vi "WS1050 36 DUT Reliability HD_Cycling Ver1.6.vi"() -> ()   [LabVIEW 2012]
uses:
  WS_VCAP Driver 029/Source/WSVCAP Shell/Type Defs/WSVCAP SHL I2C DUT Mask Mode Enum.ctl
  <vilib>/Utility/file.llb/Read From Spreadsheet File (DBL).vi
panel:
  out "VISA resource name out":refnum<visa-resource-name>="GPIB0::3::INSTR"
  out "error out 2":errorcluster={"status"=TRUE, "code"=-63192, "source"="niLvFpga_Open_PXI-7813R.vi"}
  in  "Reg1_Bit Cntrl":string[](array[string])=["01", "02", "04", "08", "10", "20", "40", "80", "03", "06", "0C", "D8", "33", "66", "CC", "07", "0E", "1C", "38", "70", "E0", "0F", "1E", "3C", "78", "F0", "1F", "3E", "7C", "F8", "3F", "7E", "FC", "7F", "FE", "FD", "FB", "F7", "EF", "DF", "BF", "7F", "FC", "F9", "F3", "E7", "CF", "9F", "3F", "F8", "F1", "E3", "C7", "8F", "1F", "F0", "E1", "C3", "87", "0F", "E0", "C1", "83", "07", "C0", "81", "03", "AA", "55", "00"]
  out "date string":string="5/19/2014"
  out "PS1 Out":refnum<visa-resource-name>
  out "Ke2000 Out":refnum<visa-resource-name>="GPIB0::9::INSTR"
  in  "VPI_Cmd":string[](array[string])=["00", "3B", "00"]
  in  "VPI Name":string[](array[string])=["All_Drivers OFF", "All Drivers ON", "All Drivers OFF2"]
  in  "Tab Control":T1(tab)
  in  "CP with DVA ON":i32(ring) items=["CP HDC 35V", "CP HDC 40.25V", "CP HDC 27.5V", "CP HDC 30.5V", "CP HDC 44V", "CP HDC 50V", "CP HDC 55V", "CP HDC 42.5V", "CP HDC 32V"]
  in  "No of Cmd":i64=2
  in  "Board#":string="BRD5"
  in  "Serial Number":string[][](table)=[["DUT", "SN"], ["DUT1", "1"], ["DUT2", "2"], ["DUT3", "3"], ["DUT4", "4"], ["DUT5", "5"], ["DUT6", "6"], ["DUT7", "7"], ["DUT8", "8"], ["DUT9", "9"], ["DUT10", "10"], ["DUT11", "11"], ["DUT12", "12"], ["DUT13", "13"], ["DUT14", "14"], ["DUT15", "15"], ["DUT16", "16"], ["DUT17", "17"], ["DUT18", "18"], ["DUT19", "19"], ["DUT20", "20"], ["DUT21", "21"], ["DUT22", "22"], ["DUT23", "23"], ["DUT24", "24"], ["DUT25", "25"], ["DUT26", "26"], ["DUT27", "27"], ["DUT28", "28"], ["DUT29", "29"], ["DUT30", "30"], ["DUT31", "31"], ["DUT32", "32"], ["DUT33", "33"], ["DUT34", "34"], ["DUT35", "35"], ["DUT36", "36"]]
  in  "SPI Clock Rate (Hz)":dbl=5000000.0 caption="Cycle Speed" format="%.1p Hz"
  in  "Wafer#":string="T7-EB"
  in  "File Name":string="CYC_WS1050_T7_EB_65C_40V_25DC_EMPTY_BRD5_151017_1"
  in  "TMN DC\\CAP Data Log File Path":path=path "C:/WS1050 36 DUT Data"
  in  "Test Program":string="WS1050 36 DUT Reliability HD_Cycling Ver1.5"
  out "Current Date":string="8/28/2014"
  out "Current Time":string="0950"
  in  "Start Date":string="10/21/2014"
  in  "Start Time":string="1542"
  in  "Comment":string="CYC65C40V"
  in  "OK Button":bool
  in  "Calibration":bool
  in  "Verify CP":bool
  in  "CP Setting":i32(ring) items=["CP OFF", "CP ON", "CP 35V", "CP 40V", "DVA ON", "DVA OFF", "REG1 ON", "REG1 OFF", "REG2 ON", "REG2 OFF", "REG3 ON", "REG3 OFF"]
  in  "Set VDD":dbl=3.7 format="%.3g"
  in  "Command":string[](array[string])=["0702013B3B3B", "070201000000", "0702013B0000"]
  in  "Clock Rate (Hz)":dbl=1000000.0 caption="Meas Speed" format="%.1p Hz"
  out "AR  Measurent(Hz)":dbl
  in  "PS1 Source":refnum<visa-resource-name>="GPIB0::5::INSTR"
  in  "Ke2000":refnum<visa-resource-name>="GPIB0::9::INSTR"
  in  "CP to HD/Cycle":i32(ring)=1 items=["CP HDC 35V", "CP HDC 40.25V", "CP HDC 27.5V", "CP HDC 30.5V", "CP HDC 44V", "CP HDC 50V", "CP HDC 55V", "CP HDC 42.5V", "CP HDC 32V"]
  out "Simulate FPGA":bool
  out "Online":bool
  out "AR Cycling(Hz)":dbl=5000000.0
  in  "Ke2400":refnum<visa-resource-name>="GPIB0::3::INSTR"
  in  "Initialize AD7747":bool
  in  "DUT Mask Mode":T2=enum."All"
  in  "RFFE Slave Address":u8=7 caption="Slave Address" format="0x%02x"
  out "Activity Log":string="05/19/2014 -- 12:24:35.853::WSVCAP::APP::Application Started\n05/19/2014 -- 12:24:37.606::WSVCAP::WSVCAP SHL::WR I2C-REG:0x0A;MASK:0xFFFFFFFFFFFF;C1 DATA:22:22:22:22:22:22:22:22:22:22:22:22:22:22:22:22;C2 DATA:22:22:22:22:22:22:22:22:22:22:22:22:22:22:22:22;C3 DATA:22:22:22:22:22:22:22:22:22:22:22:22:22:22:22:22\r\n05/19/2014 -- 12:24:37.773::WSVCAP::WSVCAP SHL::WR I2C-ST:0,0,4,1\r\n05/19/2014 -- 12:24:37.903::WSVCAP::WSVCAP SHL::RD I2C-BYTES:4;ADD:0x00;MASK:0xFFFFFFFFFFFF\r\n05/19/2014 -- 12:24:38.045::WSVCAP::WSVCAP SHL::RD I2C:C1 DATA:2:2:2:2:2:2:2:2:2:2:2:2:2:2:2:2|A7:A9:AA:82:82:7F:82:81:82:81:83:82:81:82:82:81|46:36:BB:88:44:A3:E9:2B:32:20:ED:25:BB:3D:68:B|2C:6A:EB:A7:22:56:FE:CC:36:82:D7:B0:3B:48:F9:CC;C2 DATA:2:2:2:2:2:2:2:2:2:2:2:2:2:2:2:2|94:94:94:80:80:80:80:80:81:7E:7E:81:80:7E:80:80|47:33:15:82:62:B:E8:1C:D7:C3:7D:41:7C:B7:4C:2A|C4:B4:AE:8:1E:D1:4E:37:11:C0:6F:63:42:9D:63:B5;C3 DATA:2:2:2:2:2:2:2:2:2:2:2:2:2:2:2:2|95:95:95:81:81:7E:81:80:84:7D:80:83:81:7E:7F:80|AB:C4:14:B5:7B:52:DF:C9:79:5D:5F:30:99:31:1E:F4|6E:5C:F7:A8:C3:EB:7B:EF:33:92:89:77:4D:67:75:DD;STATUS:0:0:4:0\r\n05/19/2014 -- 12:24:38.046::WSVCAP::WSVCAP SHL::WR I2C-REG:0x0A;MASK:0xFFFFFFFFFFFF;C1 DATA:22:22:22:22:22:22:22:22:22:22:22:22:22:22:22:22;C2 DATA:22:22:22:22:22:22:22:22:22:22:22:22:22:22:22:22;C3 DATA:22:22:22:22:22:22:22:22:22:22:22:22:22:22:22:22\r\n05/19/2014 -- 12:24:38.089::WSVCAP::WSVCAP SHL::WR I2C-ST:0,0,4,1\r\n05/19/2014 -- 12:24:38.219::WSVCAP::WSVCAP SHL::RD I2C-BYTES:4;ADD:0x00;MASK:0xFFFFFFFFFFFF\r\n05/19/2014 -- 12:24:38.362::WSVCAP::WSVCAP SHL::RD I2C:C1 DATA:2:2:2:2:2:2:2:2:2:2:2:2:2:2:2:2|A7:AB:AA:82:82:82:83:83:82:82:82:82:7F:82:82:81|4B:32:96:83:3E:61:43:17:25:62:AB:4D:A2:40:2E:5|3C:76:2B:B4:EE:E4:A9:1A:AA:A:26:C7:21:2E:87:5B;C2 DATA:2:2:2:2:2:2:2:2:2:2:2:2:2:2:2:2|94:94:94:80:80:80:80:80:80:7F:80:81:80:80:7F:80|4A:32:19:7D:19:6C:79:46:61:7F:4B:B8:A5:30:F3:14|B4:70:A:8C:9C:DC:43:FA:1E:A:C6:21:A:A9:13:F3;C3 DATA:2:2:2:2:2:2:2:2:2:2:2:2:2:2:2:2|95:97:94:81:80:81:82:81:80:7E:81:84:7F:81:80:80|B2:32:D0:A7:9E:4C:AB:D4:EE:D9:F0:82:B7:91:7:FF|C1:91:B6:3D:D8:E:1B:4F:9F:6A:F1:6C:E7:3F:7:BA;STATUS:0:0:4:0\r\n05/19/2014 -- 12:24:38.364::WSVCAP::WSVCAP SHL::WR I2C-REG:0x0A;MASK:0xFFFFFFFFFFFF;C1 DATA:22:22:22:22:22:22:22:22:22:22:22:22:22:22:22:22;C2 DATA:22:22:22:22:22:22:22:22:22:22:22:22:22:22:22:22;C3 DATA:22:22:22:22:22:22:22:22:22:22:22:22:22:22:22:22\r\n05/19/2014 -- 12:24:38.406::WSVCAP::WSVCAP SHL::WR I2C-ST:0,0,4,1\r\n05/19/2014 -- 12:24:38.536::WSVCAP::WSVCAP SHL::RD I2C-BYTES:4;ADD:0x00;MASK:0xFFFFFFFFFFFF\r\n05/19/2014 -- 12:24:38.678::WSVCAP::WSVCAP SHL::RD I2C:C1 DATA:2:2:2:2:2:2:2:2:2:2:2:2:2:2:2:2|A7:A9:AB:82:82:81:82:82:82:82:82:82:82:82:82:81|46:71:4C:87:43:3D:7F:FC:25:4F:8E:54:97:3E:60:8C|AA:F4:1F:B5:CE:43:1F:36:9:87:9C:78:86:5:B6:8E;C2 DATA:2:2:2:2:2:2:2:2:2:2:2:2:2:2:2:2|94:94:94:80:7F:7F:80:80:80:80:80:81:80:80:80:80|49:36:18:7D:6E:C5:E4:3C:81:2E:41:D3:75:71:E3:72|E8:D3:E6:D1:E0:48:AE:D4:54:D:E8:8E:B4:41:68:4;C3 DATA:2:2:2:2:2:2:2:2:2:2:2:2:2:2:2:2|95:95:95:81:7F:7F:81:81:81:81:81:84:81:81:82:81|B3:F5:90:AB:82:69:7B:93:D0:77:E8:D5:E8:8C:84:E8|B9:AC:EE:2B:B6:71:8F:4A:74:31:56:BB:8A:B7:A0:C8;STATUS:0:0:4:0\r\n05/19/2014 -- 12:24:38.681::WSVCAP::WSVCAP SHL::WR I2C-REG:0x0A;MASK:0xFFFFFFFFFFFF;C1 DATA:22:22:22:22:22:22:22:22:22:22:22:22:22:22:22:22;C2 DATA:22:22:22:22:22:22:22:22:22:22:22:22:22:22:22:22;C3 DATA:22:22:22:22:22:22:22:22:22:22:22:22:22:22:22:22\r\n05/19/2014 -- 12:24:38.723::WSVCAP::WSVCAP SHL::WR I2C-ST:0,0,4,1\r\n05/19/2014 -- 12:24:38.854::WSVCAP::WSVCAP SHL::RD I2C-BYTES:4;ADD:0x00;MASK:0xFFFFFFFFFFFF\r\n05/19/2014 -- 12:24:38.996::WSVCAP::WSVCAP SHL::RD I2C:C1 DATA:2:2:2:2:2:2:2:2:2:2:2:2:2:2:2:2|A7:A9:AA:82:82:7F:83:81:82:81:84:82:7F:82:7F:82|43:FB:E:7F:3C:AD:35:35:26:A2:6C:21:4B:3D:8:6|63:9A:E1:F3:95:32:91:42:90:3C:78:1F:5C:D7:5F:D8;C2 DATA:2:2:2:2:2:2:2:2:2:2:2:2:2:2:2:2|94:94:94:80:80:80:80:80:81:80:7E:81:80:7E:7F:80|48:36:18:7F:5E:3D:69:83:DE:AE:A1:9E:31:AE:BB:96|15:A0:44:17:13:FD:CC:C8:6D:B2:EF:A7:C:C7:3B:F;C3 DATA:2:2:2:2:2:2:2:2:2:2:2:2:2:2:2:2|95:96:94:81:81:7E:82:80:84:80:80:84:7F:7E:7D:82|AD:3B:6D:A9:7C:57:9D:F5:7A:96:23:5C:36:2D:ED:5A|CD:46:DB:3B:C7:BD:70:60:33:B8:B:F7:63:A:51:4D;STATUS:0:0:4:0\r\n05/19/2014 -- 12:24:38.998::WSVCAP::WSVCAP SHL::WR I2C-REG:0x0A;MASK:0xFFFFFFFFFFFF;C1 DATA:22:22:22:22:22:22:22:22:22:22:22:22:22:22:22:22;C2 DATA:22:22:22:22:22:22:22:22:22:22:22:22:22:22:22:22;C3 DATA:22:22:22:22:22:22:22:22:22:22:22:22:22:22:22:22\r\n05/19/2014 -- 12:24:39.040::WSVCAP::WSVCAP SHL::WR I2C-ST:0,0,4,1\r\n05/19/2014 -- 12:24:39.170::WSVCAP::WSVCAP SHL::RD I2C-BYTES:4;ADD:0x00;MASK:0xFFFFFFFFFFFF\r\n05/19/2014 -- 12:24:39.311::WSVCAP::WSVCAP SHL::RD I2C:C1 DATA:2:2:2:2:2:2:2:2:2:2:2:2:2:2:2:2|A7:AA:AB:82:82:81:82:81:82:81:82:82:82:82:7F:82|44:F1:90:87:45:44:C8:2C:2C:F1:FC:1B:94:3B:3C:75|4A:49:95:19:99:73:64:3:23:24:F3:A2:5E:7F:C4:B6;C2 DATA:2:2:2:2:2:2:2:2:2:2:2:2:2:2:2:2|94:94:94:80:80:80:80:7F:80:80:7E:80:80:7E:7F:80|4C:36:17:7D:A8:9F:DE:C7:53:6D:8A:F4:41:A5:C6:E0|90:2E:24:C:D9:22:E4:76:3B:40:1D:53:33:B1:3E:4D;C3 DATA:2:2:2:2:2:2:2:2:2:2:2:2:2:2:2:2|95:97:95:81:81:7F:81:80:80:81:7F:82:81:7E:7D:82|AE:2B:A7:AB:CC:CD:A4:38:FD:17:80:F2:92:2D:45:C4|76:E5:D:B9:AD:B5:BA:8D:28:32:9E:42:B7:20:4A:D9;STATUS:0:0:4:0\r\n05/19/2014 -- 12:24:39.313::WSVCAP::WSVCAP SHL::WR I2C-REG:0x0A;MASK:0xFFFFFFFFFFFF;C1 DATA:22:22:22:22:22:22:22:22:22:22:22:22:22:22:22:22;C2 DATA:22:22:22:22:22:22:22:22:22:22:22:22:22:22:22:22;C3 DATA:22:22:22:22:22:22:22:22:22:22:22:22:22:22:22:22\r\n05/19/2014 -- 12:24:39.355::WSVCAP::WSVCAP SHL::WR I2C-ST:0,0,4,1\r\n05/19/2014 -- 12:24:39.486::WSVCAP::WSVCAP SHL::RD I2C-BYTES:4;ADD:0x00;MASK:0xFFFFFFFFFFFF\r\n05/19/2014 -- 12:24:39.628::WSVCAP::WSVCAP SHL::RD I2C:C1 DATA:2:2:2:2:2:2:2:2:2:2:2:2:2:2:2:2|A7:A9:AA:82:82:82:83:82:82:82:82:82:7F:82:7F:82|47:18:E4:87:3E:E7:6:65:25:92:37:38:A8:3E:89:85|7C:A7:7:2B:A3:7A:EC:EF:89:ED:F4:D3:D8:BC:3A:F5;C2 DATA:2:2:2:2:2:2:2:2:2:2:2:2:2:2:2:2|94:94:94:80:7F:80:80:7F:81:80:7E:80:80:80:81:80|49:37:17:80:76:25:6A:F8:DF:55:97:4D:B8:5B:2B:B1|13:E3:9A:3E:1A:2D:4F:B6:DB:E9:61:FA:8B:D6:9:CC;C3 DATA:2:2:2:2:2:2:2:2:2:2:2:2:2:2:2:2|95:95:95:81:7F:80:82:81:84:80:7F:81:80:81:7F:82|AF:93:3B:AF:5B:11:82:E4:7E:C3:2D:72:9:96:D9:A|DB:96:F2:10:5F:64:9A:C6:98:12:27:7D:10:D3:20:D9;STATUS:0:0:4:0\r\n05/19/2014 -- 12:24:40.132::WSVCAP::WSVCAP SHL::CLOSE\r\n"
  in  "C1 Cap DAC":u8=128 caption="B Data In" format="0x%02x"
  in  "C2 Cap DAC":u8=128 caption="B Data In" format="0x%02x"
  in  "C3 Cap DAC":u8=128 caption="B Data In" format="0x%02x"
  out "IDD Brd(uA)":string
  in  "Repeat Meas(s)":u32=900
  in  "Real No. From\nLookup Table":bool
  in  "Control Panel":T3={"Verify Socket"=FALSE, "HD/CYC"=FALSE, "E-CAL"=FALSE, "DVA"=FALSE, "VPI"=TRUE, "VSA"=TRUE, "HS"=TRUE}
  out "Verify Socket":bool
  out "HD/CYC":bool
  out "E-CAL":bool
  out "DVA":bool
  out "VPI":bool
  out "VSA":bool
  out "HS":bool
  in  "Lot#":string="WS1050"
  out "AD7747 Values":string[][](table)
  in  "Freq(Hz)":string="12K"
  in  "Reset P/S":bool
  in  "Test Sequences":i32(ring) items=["C1_C2_C3", "C2_C1_C3", "C3_C2_C1"]
  in  "WS1050/51":bool=TRUE
  in  "% Duty Cycle":string="25"
  in  "Cmd To HD":string="0702013B3B3B"
  in  "Post CMd Delay":dbl[](array[numeric])=[1.7e-05, 5.4e-05, 1.8e-05] min=0.0 max=0.5 format="%#.0p s"
  in  "Cmin/Act":bool=TRUE
  in  "CP to Meas":i32(ring)=1 items=["CP HDC 35V", "CP HDC 40.25V", "CP HDC 27.5V", "CP HDC 30.5V", "CP HDC 44V", "CP HDC 50V", "CP HDC 55V", "CP HDC 42.5V", "CP HDC 32V"]
  in  "CP VPI":i32(ring) items=["CP HDC 35V", "CP HDC 40.25V", "CP HDC 27.5V", "CP HDC 30.5V", "CP HDC 44V", "CP HDC 50V", "CP HDC 55V", "CP HDC 42.5V", "CP HDC 32V"]
  out "CAP_C1":string[][](table)
  out "NOM IDD OFF(uA)":string
  out "CAP_C2":string[][](table)
  out "CAP_C3":string[][](table)
  out "Total Time":u64
  in  "Set HD/Cycle \nto Complete":u64=5000000000
  out "No of HD/Cycle\nCompleted":u64
  out "Cycle Count":u64 min=1 max=4 step=1
  out "Loop \ncompleted":i32=1
  out "Previous Time":string="12:20:26 PM"
  out "STATUS":string="Idle...."
  out "Total Delta C2(pF)":string[](array[string])
  out "Total Delta C1(pF)":string[](array[string])
  out "Total Delta C3(pF)":string[](array[string])
  out "RB Reg for HD":string[](array[string])
  out "RB Reg for HD/Cycle":string[](array[string])
  out "VPI C2":string[][](table)
  out "VPI C3":string[][](table)
  out "NOM IDD ON (uA)":string
  out "IDD_HD/CYC (uA)":string="164.601255E+0"
  in  "stop During HD/Cycles":bool
  in  "stop":bool
  out "IDD Stdby(uA)":string="2.606990E+0"
  out "VPI C1":string[][](table)
  out "VSA_V1":string[][](table)
  out "VSA_V2":string[][](table)
  out "VSA_V3":string[][](table)
  in  "VSA Voltage(V)":dbl[](array[numeric])=[-10.0, 0.0, 10.0]
  in  "DC_Temp":i32=65
  in  "HD/CYC Temp":i32=65
  in  "Time All ON (s)":u32=120
  in  "Time All OFF (s)":u32=120
  in  "HD_DC (Min)":u64=259200
  out "LPs Count":i32
  in  "X Repeat":i32=100
  out "No LPs to RP":i32
  out "Run Loops":i32=1
  out "TTCompleted":u64=2000
  in  "TTF Completed":u64=5000000000
  out "% Delta C_T0":string[][](array[string])
  out "% Delta C":string[][](array[string])
  out "EFuse RB T0":string[](array[string])
  out "Current EFuse Read back":string[](array[string])
  out "EFuse Readback Status":bool[](array[boolean])
  in  "DeltaC Target Setting(pF)":dbl=7.375
  out "error out":errorcluster
  in  "error in (no error)":errorcluster
  in  "HD RP":dbl=60.0
  in  "Cycle RP":dbl=10000.0
  out "Min Plot_1":dbl[][](graph) caption="(Y) Multi Plot 2"
  out "Min Plot_2":dbl[][](graph) caption="(Y) Multi Plot 2"
  out "Min Plot_3":dbl[][](graph) caption="(Y) Multi Plot 2"
  in  "Debug":bool
  in  "No of Rows\nFrom Spread Sheet":i32
  in  "Plot Delta Cmin":bool=TRUE
  in  "Plot":T4(ring)
  in  "Bank C1":i32(ring) items=["C1", "C2", "C3", "D_C1", "D_C2", "D_C3"]
  in  "Bank C2":i32(ring)=1 items=["C1", "C2", "C3", "D_C1", "D_C2", "D_C3"]
  in  "Bank C3":i32(ring)=2 items=["C1", "C2", "C3", "D_C1", "D_C2", "D_C3"]
  # "Company:  WiSpry Inc\n20 Fairbanks Ste 198 Irvine CA 92618\n\nAuthor:  Andy V Tran\nCreated:  09/10/2015\nLabVIEW 2012 Pro\nTest Program:  WS1050 36 DUT Reliability HD_Cycling ver1.6\nFPGA: WS_VCAP Driver 029"
  # "Note for HD Duty Cycle:\n1.  Set time to start HD_DC (Min), = 6 or 24 hrs; default is 259200 (6 months) \n2.  Set Time for HD_CYC ON/OFF, default setting is 2 Min ON + 2 Min OFF with specific time.  Normally is 48hrs.\n3.  Set HD/Cycle to completed = item 1 + item 2 = 6 or 24hrs + 48 hrs\n4.  Set X Repeat = number of runs, default is 100 runs; each run is = item 3\n5.  Set TTF Completed to stop the test.\n\nVer 1.5 updated based on Ver1.4:\n1.  Updated calibration procedure by changing offset cal in series"
  # "Minutes"
  # "X1000"
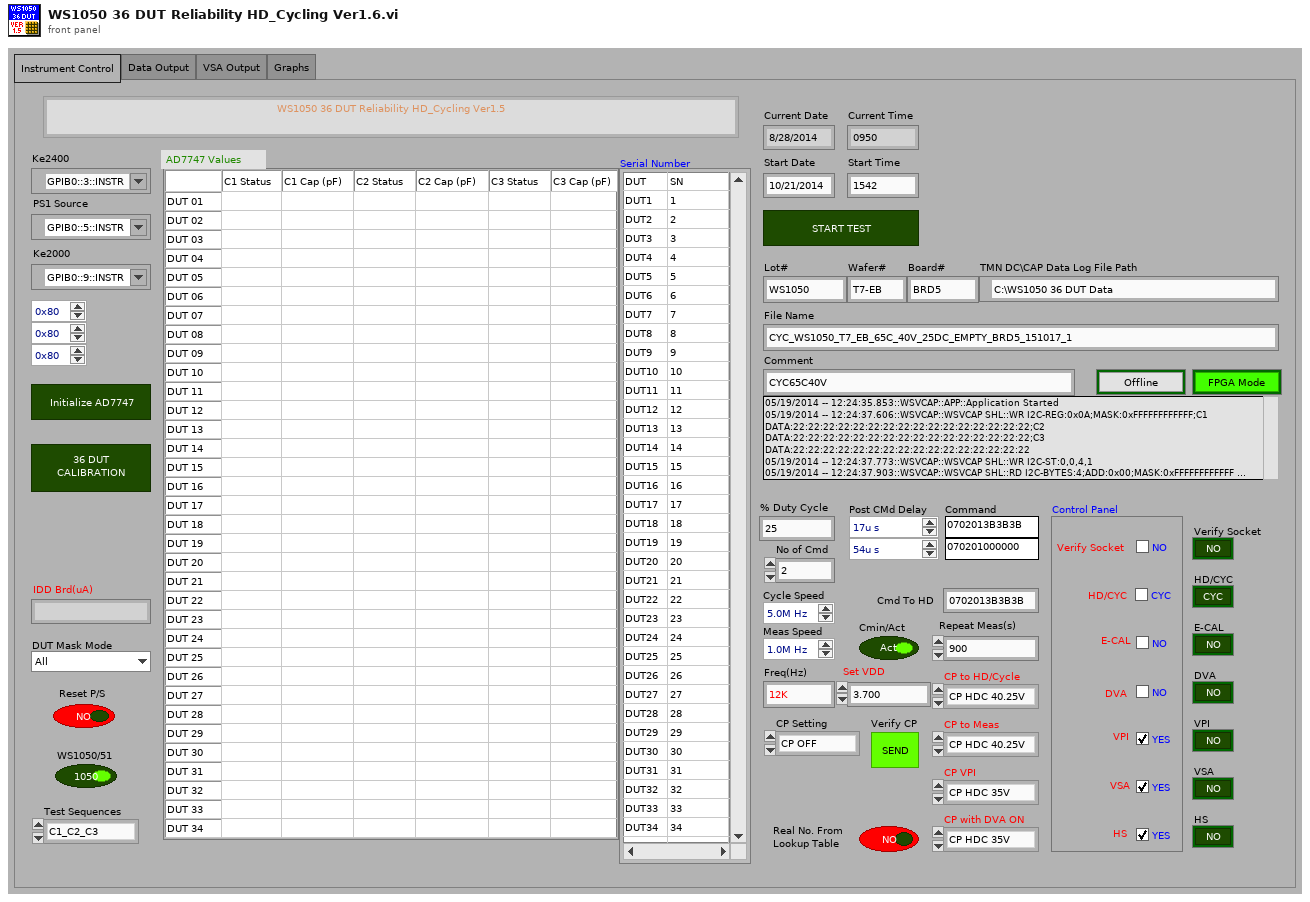
[diagram p1: front panel]
types:
  T1 = enum32{"Instrument Control", "Data Output", "VSA Output", "Graphs"}
  T2 = typedef "WSVCAP SHL I2C DUT Mask Mode Enum.ctl" = enum16{"Custom", "C1", "C2", "C3", "All"}
  T3 = cluster{"Verify Socket":bool, "HD/CYC":bool, "E-CAL":bool, "DVA":bool, "VPI":bool, "VSA":bool, "HS":bool}
  T4 = enum16{"ALL DUTs", "DUT 01", "DUT 02", "DUT 03", "DUT 04", "DUT 05", "DUT 06", "DUT 07", "DUT 08", "DUT 09", "DUT 10", "DUT 11", "DUT 12", "DUT 13", "DUT 14", "DUT 15", "DUT 16", "DUT 17", "DUT 18", "DUT 19", "DUT 20", "DUT 21", "DUT 22", "DUT 23", "DUT 24", "DUT 25", "DUT 26", "DUT 27", "DUT 28", "DUT 29", "DUT 30", "DUT 31", "DUT 32", "DUT 33", "DUT 34", "DUT 35", "DUT 36"}
  T5 = typedef "WSVCAP SHL Core System Cluster.ctl" = cluster{"Settings":T6, "FPGA Resource":tag, "Online":bool, "I2C Wait Ticks":u32, "SPI Wait Ticks":u32, "RFFE Wait Ticks":u32}
  T6 = typedef "WSVCAP SHL I2C Settings Cluster.ctl" = cluster{"FPGA Resource Name":string, "I2C Slave Address":u8, "I2C Clock Rate (Hz)":dbl, "SPI Clock Rate (Hz)":dbl, "RFFE Slave Address":u8, "RFFE Clock Rate (Hz)":dbl, "Simulate FPGA":bool, "C1 Cap DAC Default":u8, "C2 Cap DAC Default":u8, "C3 Cap DAC Default":u8}
  T7 = enum16{"Idle...", "Voltage 1", "Voltage 2", "Voltage 3"}[]
  T8 = cluster{"Test Program ":string, "Comment":string, "Data Out":string, "Data Out":string, "Data Out":string, string, "Data Out":string, "Data Out":string, "Data Out":string, "Freq(Hz)":string, "Board#":string}
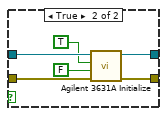
[diagram p2: hidden frame]
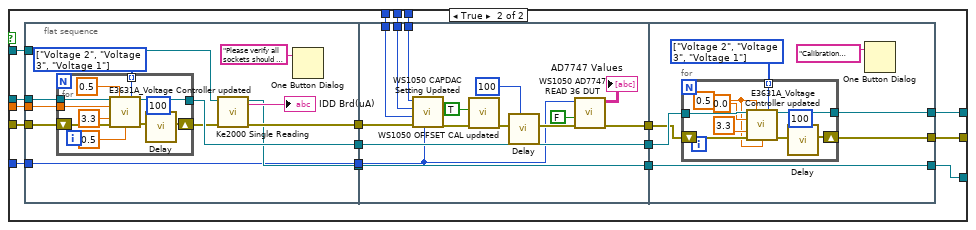
[diagram p10: hidden frame]
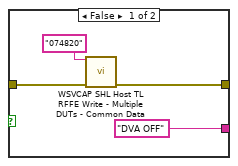
[diagram p11: hidden frame]
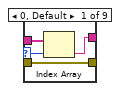
[diagram p12: hidden frame]
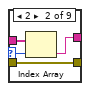
[diagram p13: hidden frame]
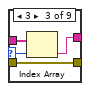
[diagram p14: hidden frame]
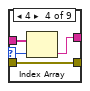
[diagram p15: hidden frame]
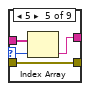
[diagram p16: hidden frame]
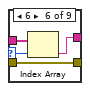
[diagram p17: hidden frame]
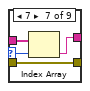
[diagram p18: hidden frame]
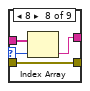
[diagram p19: hidden frame]
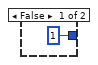
[diagram p20: hidden frame]
diagram:
  w25 = TRUE
  w29 = u16 0 items=["Off", "Moving Filter", "Repeating Filter"] ("Digital Filter (0: Off)")
  w30 = u16 7 items=["3.5 Digits"=4, "4.5 Digits"=5, "5.5 Digits"=6, "6.5 Digits"=7] ("Resolution (7: 6.5 digits)")
  n1 = case shown="True" w25 {
    tunnel: "error in (no error)" -> [w37 w38]
    tunnel: [w37 w45] -> w14
    frame False {
    }
    frame True {
      n2 = call "WSVCAP SHL Host TL Initialize.vi"("error in"=w38) -> ("error out"=w39:errorcluster)  [unwired: 13 in, 1 out]
      n3 = control-ref of="Activity Log"() -> (w41:refnum<vi>)
      n4 = call "ACT LG Activity Log Core.vi"("Display Ref"=w41, "Source"="WSVCAP", "Error In (no error)"=w39) -> ("Error Out"=w40:errorcluster)  [unwired: 11 in, 1 out]
      n5 = call "WSVCAP SHL Host TL Status Manager.vi"("error in"=w40) -> ("System Out"=w46:T5, "error out"=w45:errorcluster)  [unwired: 13 in]
      n6 = Unbundle By Name(w46) -> ("Online"=→"Online":bool, "Settings.Simulate FPGA"=→"Simulate FPGA":bool)
    }
  }
  n7 = case shown="True" TRUE {
    tunnel: w14 -> [w47 w52]
    tunnel: [w48 w51] -> w22
    tunnel: [w47 w50] -> w18
    tunnel: "Ke2400" -> [w48 w49]
    frame False {
    }
    frame True {
      n8 = VISA Write(VISA resource name=w49, write buffer="SOUR:FUNC VOLT;VOLT:MODE FIX;RANG 100;LEV 0.0;:SENS:FUNC \"CURR\";CURR:PROT 60E-3;RANG 100E-3;:OUTP ON", error in (no error)=w52) -> (VISA resource name out=w51:refnum<visa-resource-name>, error out=w50:errorcluster)  [unwired: 1 out]
    }
  }
  n9 = case shown="False" "Reset P/S" {
    tunnel: "PS1 Source" -> [w54 w61]
    tunnel: [w54 w59] -> w34
    tunnel: w14 -> [w55 w57]
    tunnel: [w55 w56] -> w13
    frame False {
    }
    frame True {
      n10 = call "Agilent 3631A Initialize.vi"("error in (no error)"=w57, "Default"=FALSE ("Reset? (T: Yes)"), "Reset"=TRUE ("ID Query? (T: Yes)"), "VISA resource name"=w61) -> ("error out"=w56:errorcluster, "VISA resource name out"=w59:refnum<visa-resource-name>)  [unwired: 6 in]
    }
  }
  n11 = call "Ke2000 Initialize.vi"("error in (no error)"=w14, "VISA resource name"="Ke2000") -> ("error out"=w31:errorcluster, "VISA resource name out"=w32:refnum<visa-resource-name>)  [unwired: 8 in]
  n12 = call "Ke2000 Configure DC Current.vi"("Resolution (7: 6.5 digits)"=w30, "Digital Filter (0: Off)"=w29, "Auto Range? (T: Auto)"=FALSE, "error in"=w31, "Custom Range (0 A)"=1.0, "VISA resource name"=w32) -> ("error out"=w15:errorcluster, "VISA resource name out"=w27:refnum<visa-resource-name>)  [unwired: 4 in]
  n13 = case shown="True" TRUE {
    tunnel: [_ w62] -> w36
    frame False {
    }
    frame True {
      n14 = call-poly <vilib>:"Read From Spreadsheet File.vi"("number of rows (all:-1)"=-1) -> ("all rows"=w62:dbl[][])  [unwired: 6 in, 4 out]
    }
  }
  n15 = Merge Errors(w18, w15, w13) -> (w23:errorcluster)
  n16 = while {
    tunnel: w23 -> [w70]
    tunnel: [w66] -> w4
    tunnel: w36 -> [w93]
    tunnel: w34 -> [w81]
    tunnel: w27 -> [w82]
    tunnel: [w91] -> w10
    tunnel: [w90] -> w5
    tunnel: w22 -> [w88]
    tunnel: [w87] -> w20
    tunnel: [FALSE ("stop")] -> w16
    i -> [w89]
    stop <- w94 stop-if-true
    n17 = case shown="0" w89 {
      tunnel: w70 -> [w104 w106]
      tunnel: [w103 w106] -> w84
      tunnel: "RFFE Slave Address" -> [w101 _]
      frame 0 {
        w97 = dbl[][] []
        w96 = "" ("uA")
        w98 = string[][] []
        w99 = string[] [] ("EFuse Read back")
        w105 = u64 0 ("No of HD/Cycle\nCompleted")
        n18 = local write "RB Reg for HD/Cycle"(w99) -> ()
        n19 = local write "Current EFuse Read back"(w99) -> ()
        n20 = local write "EFuse RB T0"(w99) -> ()
        n21 = local write "Total Delta C1(pF)"(w99) -> ()
        n22 = local write "Total Delta C2(pF)"(w99) -> ()
        n23 = local write "Total Delta C3(pF)"(w99) -> ()
        n24 = local write "No of HD/Cycle\nCompleted"(w105) -> ()
        n25 = local write "Cycle Count"(w105) -> ()
        n26 = local write "CAP_C2"(w98) -> ()
        n27 = local write "CAP_C1"(w98) -> ()
        n28 = local write "VPI C2"(w98) -> ()
        n29 = local write "VSA_V3"(w98) -> ()
        n30 = local write "VSA_V1"(w98) -> ()
        n31 = local write "NOM IDD OFF(uA)"(w96) -> ()
        n32 = local write "NOM IDD ON (uA)"(w96) -> ()
        n33 = local write "IDD Brd(uA)"(w96) -> ()
        n34 = local write "VSA_V2"(w98) -> ()
        n35 = local write "CAP_C3"(w98) -> ()
        n36 = local write "VPI C1"(w98) -> ()
        n37 = local write "VPI C3"(w98) -> ()
        n38 = local write "% Delta C"(w98) -> ()
        n39 = local write "% Delta C_T0"(w98) -> ()
        n40 = call "WSVCAP SHL Host TL RFFE Configure.vi"("RFFE Slave Address"=w101, "Clock Rate (Hz)"="Clock Rate (Hz)", "error in"=w104) -> ("Actual Rate (Hz)"=→"AR  Measurent(Hz)":dbl, "error out"=w103:errorcluster)  [unwired: 11 in]
        n41 = local write "Min Plot_3"(w97) -> ()
        n42 = local write "Min Plot_1"(w97) -> ()
        n43 = local write "Min Plot_2"(w97) -> ()
      }
      frame 1, Default {
      }
    }
    n44 = while {
      tunnel: ["stop"] -> w86
      tunnel: w84 -> [w137]
      tunnel: [w130] -> w78
      tunnel: w81 -> [w136]
      tunnel: w82 -> [w132]
      tunnel: [w133] -> w80
      tunnel: [w131] -> w79
      tunnel: [w128] -> w77
      tunnel: [w127] -> w76
      tunnel: [w126] -> w75
      tunnel: [w125] -> w74
      tunnel: [w124] -> w73
      tunnel: [w123] -> w72
      tunnel: [w122] -> w71
      tunnel: ["Command"] -> w69
      tunnel: ["Post CMd Delay"] -> w68
      tunnel: "Set VDD" -> [w112]
      stop <- w144 stop-if-true
      # "Set Date & Time to Start Test"
      n45 = case shown="True" "Initialize AD7747" {
        tunnel: w137 -> [w153 w159]
        tunnel: [w153 w155] -> w121
        tunnel: w136 -> [w152 w157]
        tunnel: [w152 w156] -> w135
        tunnel: w112 -> [_ w154]
        frame False {
        }
        frame True {
          w160 = T7 [enum."Voltage 2", enum."Voltage 3", enum."Voltage 1"] items=["Idle...", "Voltage 1", "Voltage 2", "Voltage 3"]
          n46 = for {
            tunnel: w157 -> [w170]
            tunnel: w160 -> [w168] mode=indexing
            tunnel: [w167] -> w156
            shift-right: [w164] -> w158
            shift-left: w159 -> [w171]
            tunnel: w154 -> [w161]
            n47 = call "E3631A_Voltage Controller updated.vi"("VISA resource name"=w170, "I_VDD(A)"=0.5, "Channel Controller"=w168, "Voltage 1"=w161, "Voltage 2"=3.3, "error in (no error)"=w171, "I_3.3V (A)"=0.5) -> ("VISA resource name out"=w167:refnum<visa-resource-name>, "error out"=w163:errorcluster)  [unwired: 7 in]
            n48 = call "Delay.vi"("milliseconds to wait"=u32 100, "error in (no error)"=w163) -> ("error out"=w164:errorcluster)  [unwired: 9 in]
          }
          n49 = call "WS1050_AD7747_Init 36DUT.vi"("error in"=w158) -> ("error out"=w155:errorcluster)  [unwired: 10 in]
        }
      }
      n50 = call "Time_stamp.vi"() -> ("date/time string"=w149:string, "date string"=w151:string)  [unwired: 2 in]
      "Current Date" <- w151
      "Current Time" <- w149
      n51 = Equal?(x=w151, y="Start Date") -> (x = y?=w147:bool)
      n52 = Equal?(x=w149, y="Start Time") -> (x = y?=w146:bool)
      n53 = And(x=w147, y=w146) -> (x .and. y?=w143:bool)
      n54 = Compound Arithmetic op=OR(w143, "OK Button", "stop") -> (w144:bool)
      n55 = case shown="False" "Calibration" {
        tunnel: w121 -> [w201 w219]
        tunnel: [w197 w216] -> w119
        tunnel: w135 -> [w200 w215]
        tunnel: [w200 w212] -> w134
        tunnel: w132 -> [w199 w211]
        tunnel: [w199 w208] -> w131
        tunnel: w112 -> [_ w207]
        tunnel: "DUT Mask Mode" -> [w196 w205]
        tunnel: "C1 Cap DAC" -> [_ w204]
        tunnel: "C2 Cap DAC" -> [_ w203]
        tunnel: "C3 Cap DAC" -> [_ w202]
        frame False {
          n56 = call "WS1050 AD7747 READ 36 DUT.vi"("error in"=w201, "Log (T)"=FALSE, "DUT Mask Mode (All)"=w196) -> ("error out"=w197:errorcluster, "AD7747 Values"=w195:string[][])  [unwired: 7 in]
          n57 = local write "AD7747 Values"(w195) -> ()
        }
        frame True {
          n58 = flat-sequence {
            tunnel: w219 -> [w230]
            tunnel: [w226] -> w218
            tunnel: w215 -> [w229]
            tunnel: [w228] -> w214
            tunnel: w211 -> [w224]
            tunnel: [w223] -> w210
            tunnel: w207 -> [w222]
            tunnel: [w221] -> w206
            tunnel: w205 -> [w221]
            tunnel: w218 -> [w255]
            tunnel: [w244] -> w217
            tunnel: w214 -> [w257]
            tunnel: [w257] -> w213
            tunnel: w210 -> [w256]
            tunnel: [w256] -> w209
            tunnel: w206 -> [w243]
            tunnel: w204 -> [w252]
            tunnel: w203 -> [w251]
            tunnel: w202 -> [w250]
            tunnel: w217 -> [w260]
            tunnel: [w263] -> w216
            tunnel: w213 -> [w262]
            tunnel: [w259] -> w212
            tunnel: w209 -> [w258]
            tunnel: [w258] -> w208
            frame #0 {
              w231 = T7 [enum."Voltage 2", enum."Voltage 3", enum."Voltage 1"] items=["Idle...", "Voltage 1", "Voltage 2", "Voltage 3"]
              n59 = for {
                tunnel: w229 -> [w241]
                tunnel: w231 -> [w239] mode=indexing
                tunnel: [w238] -> w228
                shift-right: [w236] -> w225
                shift-left: w230 -> [w242]
                tunnel: w222 -> [w232]
                n60 = call "E3631A_Voltage Controller updated.vi"("VISA resource name"=w241, "I_VDD(A)"=0.5, "Channel Controller"=w239, "Voltage 1"=w232, "Voltage 2"=3.3, "error in (no error)"=w242, "I_3.3V (A)"=0.5) -> ("VISA resource name out"=w238:refnum<visa-resource-name>, "error out"=w235:errorcluster)  [unwired: 7 in]
                n61 = call "Delay.vi"("milliseconds to wait"=u32 100, "error in (no error)"=w235) -> ("error out"=w236:errorcluster)  [unwired: 9 in]
              }
              n62 = call "Ke2000 Single Reading.vi"("error in (no error)"=w225, "VISA resource name"=w224) -> ("error out"=w226:errorcluster, "VISA resource name out"=w223:refnum<visa-resource-name>, "uA"=→"IDD Brd(uA)":string)  [unwired: 5 in, 2 out]
              n63 = One Button Dialog(message="Please verify all sockets should be empty...") -> ()  [unwired: 1 in, 1 out]
            }
            frame #1 {
              n64 = call "WS1050 CAPDAC Setting Updated.vi"("DUT Mask Mode (All)"=w243, "error in"=w255, "C3 Cap DAC"=w250, "C2 Cap DAC"=w251, "C1 Cap DAC"=w252) -> ("error out"=w253:errorcluster)  [unwired: 6 in]
              n65 = call "WS1050 OFFSET CAL updated.vi"("error in"=w253, "OFFSET CAL"=TRUE ("Read?")) -> ("error out"=w248:errorcluster)  [unwired: 9 in]
              n66 = call "Delay.vi"("milliseconds to wait"=u32 100, "error in (no error)"=w248) -> ("error out"=w247:errorcluster)  [unwired: 9 in]
              n67 = call "WS1050 AD7747 READ 36 DUT.vi"("error in"=w247, "Log (T)"=FALSE, "DUT Mask Mode (All)"=w243) -> ("error out"=w244:errorcluster, "AD7747 Values"=→"AD7747 Values":string[][])  [unwired: 7 in]
            }
            frame #2 {
              w261 = T7 [enum."Voltage 2", enum."Voltage 3", enum."Voltage 1"] items=["Idle...", "Voltage 1", "Voltage 2", "Voltage 3"]
              n68 = for {
                tunnel: w262 -> [w274]
                tunnel: w261 -> [w271] mode=indexing
                tunnel: [w270] -> w259
                shift-right: [w267] -> w263
                shift-left: w260 -> [w272]
                w265 = 0.5 ("I_VDD(A)")
                n69 = call "E3631A_Voltage Controller updated.vi"("VISA resource name"=w274, "I_VDD(A)"=w265, "Channel Controller"=w271, "Voltage 1"=0.0, "Voltage 2"=3.3, "error in (no error)"=w272, "I_3.3V (A)"=w265) -> ("VISA resource name out"=w270:refnum<visa-resource-name>, "error out"=w266:errorcluster)  [unwired: 7 in]
                n70 = call "Delay.vi"("milliseconds to wait"=u32 100, "error in (no error)"=w266) -> ("error out"=w267:errorcluster)  [unwired: 9 in]
              }
              n71 = One Button Dialog(message="Calibration Completed....") -> ()  [unwired: 1 in, 1 out]
            }
          }
        }
      }
      n72 = local write "stop During HD/Cycles"(FALSE ("stop During HD/Cycles")) -> ()
      n73 = call "Control Panel.vi"("error in (no error)"=w121, "Control Panel"="Control Panel") -> ("error out"=w118:errorcluster, "VPI"=w124:bool, "DVA"=w125:bool, "E-CAL"=w126:bool, "VSA"=w123:bool, "HD/CYC"=w127:bool, "HS"=w122:bool, "Verify Socket"=w128:bool)  [unwired: 2 in]
      "Verify Socket" <- w128
      "E-CAL" <- w126
      "VPI" <- w124
      "VSA" <- w123
      "HS" <- w122
      "HD/CYC" <- w127
      "DVA" <- w125
      n74 = Merge Errors(w118, w119) -> (w120:errorcluster)
      n75 = case shown="True" "Verify CP" {
        tunnel: [w172 w177] -> w130
        tunnel: w134 -> [w173 w180]
        tunnel: [w173 w178] -> w133
        tunnel: w120 -> [w172 w176]
        tunnel: w112 -> [_ w174]
        frame False {
        }
        frame True {
          w181 = T7 [enum."Voltage 2", enum."Voltage 3", enum."Voltage 1"] items=["Idle...", "Voltage 1", "Voltage 2", "Voltage 3"]
          # "Verify CP"
          n76 = for {
            tunnel: w180 -> [w193]
            tunnel: w181 -> [w191] mode=indexing
            shift-right: [w189] -> w179
            shift-left: w176 -> [w194]
            tunnel: [w187] -> w178
            tunnel: w174 -> [w186]
            w185 = 0.5 ("I_VDD(A)")
            n77 = call "E3631A_Voltage Controller updated.vi"("VISA resource name"=w193, "I_VDD(A)"=w185, "Channel Controller"=w191, "Voltage 1"=w186, "Voltage 2"=3.3, "error in (no error)"=w194, "I_3.3V (A)"=w185) -> ("VISA resource name out"=w187:refnum<visa-resource-name>, "error out"=w190:errorcluster)  [unwired: 7 in]
            n78 = call "Delay.vi"("milliseconds to wait"=u32 100, "error in (no error)"=w190) -> ("error out"=w189:errorcluster)  [unwired: 9 in]
          }
          n79 = Index Array(array=string[] ["074000", "074040", "07476F", "074776", "074800", "074820", "07413B", "074100", "07423B", "074200", "07433B", "074300"], index="CP Setting") -> (element=w182:string)
          n80 = call "WSVCAP SHL Host TL RFFE Write - Multiple DUTs - Common Data.vi"("Data Out"=w182, "error in"=w179, "Log (T)"=FALSE) -> ("error out"=w177:errorcluster)  [unwired: 12 in]
        }
      }
      n81 = Array Subset(array="Post CMd Delay", length="No of Cmd") -> (w116:dbl[])  [unwired: 1 in]
      n82 = Array Subset(array="Command", length="No of Cmd") -> (w117:string[])  [unwired: 1 in]
      n83 = property on="Post CMd Delay" class="Arr (strict)"("Number of Rows"="No of Cmd") -> ()  [unwired: 2 in, 2 out]
      n84 = local write "Command"(w117) -> ()
      n85 = local write "Post CMd Delay"(w116) -> ()
      n86 = property on="Command" class="Arr (strict)"("Number of Rows"="No of Cmd") -> ()  [unwired: 2 in, 2 out]
      n87 = Wait Until Next ms Multiple(millisecond multiple=u32 100) -> ()  [unwired: 1 out]
    }
    n88 = case shown="False" w86 {
      tunnel: w78 -> [w335 w1999]
      tunnel: [w320 w1999] -> w66
      tunnel: w93 -> [w336 _]
      tunnel: w80 -> [w334 w1997]
      tunnel: w79 -> [w326 w1998]
      tunnel: [w332 w1998] -> w91
      tunnel: [w330 w1997] -> w90
      tunnel: w88 -> [w323 w1996]
      tunnel: [w319 w1996] -> w87
      tunnel: "RFFE Slave Address" -> [w314 _]
      tunnel: [FALSE ("stop During HD/Cycles") FALSE ("stop During HD/Cycles")] -> _
      tunnel: w77 -> [w294 _]
      tunnel: w76 -> [w293 _]
      tunnel: w75 -> [w275 _]
      tunnel: w74 -> [w292 _]
      tunnel: w73 -> [w291 _]
      tunnel: w72 -> [w290 _]
      tunnel: w71 -> [w289 _]
      tunnel: w69 -> [w283 _]
      tunnel: w68 -> [w282 _]
      tunnel: "Set VDD" -> [w281 _]
      tunnel: [w278 FALSE ("stop During HD/Cycles")] -> w64
      frame False {
        w315 = u64 0 ("Total Completed")
        w299 = u32 100 ("milliseconds to wait")
        w331 = T7 [enum."Voltage 2", enum."Voltage 3", enum."Voltage 1"] items=["Idle...", "Voltage 1", "Voltage 2", "Voltage 3"]
        w333 = T7 [enum."Voltage 2", enum."Voltage 3", enum."Voltage 1"] items=["Idle...", "Voltage 1", "Voltage 2", "Voltage 3"]
        # "VSA"
        # "HS"
        # "HD/CYC"
        # "DVA"
        # "E-CAL"
        # "VPI"
        # "Verify Socket"
        n89 = for {
          tunnel: w335 -> [w1993]
          tunnel: w334 -> [w1992]
          tunnel: w333 -> [w1990] mode=indexing
          tunnel: [w1986] -> w328
          tunnel: [w1989] -> w318
          tunnel: w281 -> [w1983]
          n90 = call "E3631A_Voltage Controller updated.vi"("VISA resource name"=w1992, "I_VDD(A)"=0.5, "Channel Controller"=w1990, "Voltage 1"=w1983, "Voltage 2"=3.3, "error in (no error)"=w1993, "I_3.3V (A)"=0.5) -> ("VISA resource name out"=w1989:refnum<visa-resource-name>, "error out"=w1987:errorcluster)  [unwired: 7 in]
          n91 = call "Delay.vi"("milliseconds to wait"=u32 100, "error in (no error)"=w1987) -> ("error out"=w1986:errorcluster)  [unwired: 9 in]
        }
        n92 = local write "TTCompleted"(w315) -> ()
        n93 = local write "Total Time"(w315) -> ()
        n94 = call "WSVCAP SHL Host TL RFFE Write - Multiple DUTs - Common Data.vi"("Data Out"="074000", "error in"=w328, "Log (T)"=FALSE) -> ("error out"=w329:errorcluster)  [unwired: 12 in]
        n95 = local read "IDD Brd(uA)"() -> (w303:string)
        n96 = call "Delay.vi"("milliseconds to wait"=w299, "error in (no error)"=w329) -> ("error out"=w327:errorcluster)  [unwired: 9 in]
        n97 = call "Ke2000 Single Reading.vi"("error in (no error)"=w327, "VISA resource name"=w326) -> ("error out"=w304:errorcluster, "VISA resource name out"=w325:refnum<visa-resource-name>, "uA"=w306:string)  [unwired: 5 in, 2 out]
        n98 = call "Substration.vi"("error in (no error)"=w304, "Input2"=w303, "Input1"=w306) -> ("error out"=w285:errorcluster, "In1 - In2"=w305:string)  [unwired: 7 in]
        "IDD Stdby(uA)" <- w305
        n99 = case shown="True" w293 {
          tunnel: [1 ("X Repeat") w398] -> w317
          frame False {
          }
          frame True {
            n100 = local read "X Repeat"() -> (w398:i32)
          }
        }
        n101 = call "WSVCAP SHL Host TL RFFE Write - Multiple DUTs - Common Data.vi"("Data Out"="074040", "error in"=w285, "Log (T)"=FALSE) -> ("error out"=w284:errorcluster)  [unwired: 12 in]
        n102 = call "Delay.vi"("milliseconds to wait"=w299, "error in (no error)"=w284) -> ("error out"=w312:errorcluster)  [unwired: 9 in]
        n103 = case shown="True" w292 {
          tunnel: w312 -> [w349 w358]
          tunnel: [w348 w356] -> w310
          tunnel: ["DVA OFF" ("Data Out") "DVA ON" ("Data Out")] -> w311
          frame False {
            n104 = call "WSVCAP SHL Host TL RFFE Write - Multiple DUTs - Common Data.vi"("Data Out"="074820", "error in"=w349) -> ("error out"=w348:errorcluster)  [unwired: 13 in]
          }
          frame True {
            n105 = call "WSVCAP SHL Host TL RFFE Write - Multiple DUTs - Common Data.vi"("Data Out"="074800", "error in"=w358, "Log (T)"=FALSE) -> ("error out"=w354:errorcluster)  [unwired: 12 in]
            n106 = case shown="1" "CP with DVA ON" {
              selector: "CP with DVA ON" -> [w364 w368 w372 w376 w380 w384 w388 w392 w396]
              tunnel: [w363 w367 w371 w375 w379 w383 w387 w391 w394] -> w351
              tunnel: [w362 w366 w370 w374 w378 w382 w386 w390 w395] -> w353
              tunnel: w354 -> [w362 w366 w370 w374 w378 w382 w386 w390 w395]
              tunnel: string[] ["07476F", "074776", "074765", "074769", "07477B", "07477C", "07477D", "074779", "07476B"] -> [w361 w365 w369 w373 w377 w381 w385 w389 w393]
              frame 0, Default {
                n107 = Index Array(array=w361, index=w364) -> (element=w363:string)
              }
              frame 2 {
                n108 = Index Array(array=w365, index=w368) -> (element=w367:string)
              }
              frame 3 {
                n109 = Index Array(array=w369, index=w372) -> (element=w371:string)
              }
              frame 4 {
                n110 = Index Array(array=w373, index=w376) -> (element=w375:string)
              }
              frame 5 {
                n111 = Index Array(array=w377, index=w380) -> (element=w379:string)
              }
              frame 6 {
                n112 = Index Array(array=w381, index=w384) -> (element=w383:string)
              }
              frame 7 {
                n113 = Index Array(array=w385, index=w388) -> (element=w387:string)
              }
              frame 8 {
                n114 = Index Array(array=w389, index=w392) -> (element=w391:string)
              }
              frame 1 {
                n115 = Index Array(array=w393, index=w396) -> (element=w394:string)
              }
            }
            n116 = call "WSVCAP SHL Host TL RFFE Write - Multiple DUTs - Common Data.vi"("Data Out"=w351, "error in"=w353, "Log (T)"=FALSE) -> ("error out"=w356:errorcluster)  [unwired: 12 in]
          }
        }
        n117 = for {
          N: 36 -> [_]
          tunnel: "Serial Number" -> [w345]
          tunnel: [w343] -> w296 mode=indexing
          i -> [w342]
          n118 = Increment(x=w342) -> (x+1=w341:i32)
          n119 = Index Array(array=w345, index (row)=w341, index (col)=1 ("disabled index (col)")) -> (element=w343:string)
        }
        n120 = Not(x=w289) -> (.not. x?=w295:bool)
        n121 = Number To Fractional String(number=w281, precision (6)=i16 2) -> (F-format string=w308:string)  [unwired: 2 in]
        n122 = call "Delay.vi"("milliseconds to wait"=w299, "error in (no error)"=w310) -> ("error out"=w276:errorcluster)  [unwired: 9 in]
        n123 = for {
          N: w317 -> [_]
          tunnel: w336 -> [w436]
          tunnel: [w432] -> w332
          tunnel: w305 -> [w431]
          tunnel: w325 -> [w430]
          tunnel: "TMN DC\\CAP Data Log File Path" -> [w429]
          tunnel: w323 -> [w427]
          tunnel: [w426] -> w321
          tunnel: w318 -> [w403]
          shift-right: [w421] -> _
          shift-left: u64 0 -> [w423]
          tunnel: w293 -> [w420]
          tunnel: w314 -> [w415]
          tunnel: w314 -> [w414]
          tunnel: w311 -> [w413]
          tunnel: w308 -> [w412]
          tunnel: [w411] -> w302
          tunnel: w276 -> [w410]
          tunnel: w292 -> [w409]
          tunnel: w294 -> [w408]
          tunnel: w291 -> [w407]
          tunnel: w295 -> [w406]
          tunnel: w290 -> [w405]
          tunnel: w296 -> [w404]
          tunnel: [w403] -> w286
          tunnel: w283 -> [w402]
          tunnel: w282 -> [w401]
          tunnel: [w400] -> w277
          tunnel: w275 -> [w399]
          i -> [w419]
          stop <- w400 stop-if-true
          n124 = while {
            tunnel: w436 -> [w659]
            tunnel: w429 -> [w670]
            tunnel: "Lot#" -> [w669]
            tunnel: "Wafer#" -> [w668]
            tunnel: w404 -> [w667]
            tunnel: "Test Program" -> [w666]
            tunnel: w404 -> [w665]
            tunnel: "Comment" -> [w664]
            tunnel: "Lot#" -> [w663]
            tunnel: "Wafer#" -> [w662]
            tunnel: w430 -> [w658]
            tunnel: [w661] -> w432
            tunnel: w431 -> [w657]
            tunnel: w427 -> [w654]
            tunnel: [w653] -> w426
            tunnel: [w561] -> w417
            tunnel: w419 -> [w599]
            tunnel: [w590] -> w421
            tunnel: w423 -> [w589]
            shift-right: [w588] -> _
            shift-left: u64 0 -> [w487]
            tunnel: [w587] -> w416
            tunnel: w420 -> [w585]
            tunnel: w415 -> [w560]
            tunnel: w414 -> [w558]
            tunnel: w413 -> [w508]
            tunnel: w412 -> [w506]
            tunnel: [w484] -> w411
            tunnel: w410 -> [w439]
            tunnel: w409 -> [w489]
            tunnel: w408 -> [w481]
            tunnel: w407 -> [w480]
            tunnel: w406 -> [w475]
            tunnel: w405 -> [w469]
            tunnel: w402 -> [w445]
            tunnel: w401 -> [w444]
            tunnel: w399 -> [w437]
            i -> [w586]
            stop <- w600 stop-if-true
            n125 = call "WS1050 ECAL.vi"("error in (no error)"=w439, "E-CAL"=w437) -> ("error out"=w440:errorcluster, "Data Out"=w438:string)  [unwired: 8 in]
            n126 = case shown="8" "CP to HD/Cycle" {
              selector: "CP to HD/Cycle" -> [w674 w679 w684 w689 w694 w699 w704 w709 w713]
              tunnel: string[] ["07476F", "074776", "074765", "074769", "07477B", "07477C", "07477D", "074779", "07476B"] -> [w675 w680 w685 w690 w695 w700 w705 w710 w715]
              tunnel: [w673 w678 w683 w688 w693 w698 w703 w708 w714] -> w504
              tunnel: ["35.0" ("Data Out") "27.5" ("Data Out") "30.5" ("Data Out") "44.0" ("Data Out") "50.0" ("Data Out") "55.0" ("Data Out") "42.5" ("Data Out") "32.0" ("Data Out") "40.25" ("Data Out")] -> w503
              tunnel: [w671 w676 w681 w686 w691 w696 w701 w706 w711] -> w502
              tunnel: w440 -> [w671 w676 w681 w686 w691 w696 w701 w706 w711]
              frame 0, Default {
                n127 = Index Array(array=w675, index=w674) -> (element=w673:string)
              }
              frame 2 {
                n128 = Index Array(array=w680, index=w679) -> (element=w678:string)
              }
              frame 3 {
                n129 = Index Array(array=w685, index=w684) -> (element=w683:string)
              }
              frame 4 {
                n130 = Index Array(array=w690, index=w689) -> (element=w688:string)
              }
              frame 5 {
                n131 = Index Array(array=w695, index=w694) -> (element=w693:string)
              }
              frame 6 {
                n132 = Index Array(array=w700, index=w699) -> (element=w698:string)
              }
              frame 7 {
                n133 = Index Array(array=w705, index=w704) -> (element=w703:string)
              }
              frame 8 {
                n134 = Index Array(array=w710, index=w709) -> (element=w708:string)
              }
              frame 1 {
                n135 = Index Array(array=w715, index=w713) -> (element=w714:string)
              }
            }
            n136 = flat-sequence {
              tunnel: [w783] -> w652
              tunnel: [w778] -> w651
              tunnel: w659 -> [w781]
              tunnel: [w780] -> w650
              tunnel: w658 -> [w758]
              tunnel: w657 -> [w779]
              tunnel: [w779] -> w649
              tunnel: [w731] -> w648
              tunnel: [w728] -> w647
              tunnel: w502 -> [w771]
              tunnel: w599 -> [w776]
              tunnel: w586 -> [w754]
              tunnel: [w754] -> w596
              tunnel: w586 -> [w775]
              tunnel: w585 -> [w773]
              tunnel: [w772] -> w584
              tunnel: [w737] -> w579
              tunnel: [w736] -> w578
              tunnel: [w735] -> w577
              tunnel: [w741] -> w567
              tunnel: [w738] -> w566
              tunnel: w560 -> [w770]
              tunnel: [w770] -> w559
              tunnel: w558 -> [w769]
              tunnel: [w740] -> w546
              tunnel: [w739] -> w521
              tunnel: [w768] -> w509
              tunnel: w504 -> [w766]
              tunnel: [w755] -> w501
              tunnel: [w721] -> w493
              tunnel: w481 -> [w751]
              tunnel: w480 -> [w750]
              tunnel: [w750] -> w479
              tunnel: w475 -> [w749]
              tunnel: [w749] -> w474
              tunnel: w469 -> [w748]
              tunnel: [w748] -> w468
              tunnel: [w744] -> w463
              tunnel: ["Test Sequences"] -> w459
              tunnel: "Real No. From\nLookup Table" -> [w734]
              tunnel: ["WS1050/51"] -> w453
              tunnel: ["Cmin/Act"] -> w449
              tunnel: w445 -> [w723]
              tunnel: w444 -> [w722]
              tunnel: w652 -> [w1092]
              tunnel: w651 -> [w1117]
              tunnel: w650 -> [w1122]
              tunnel: [w1122] -> w557
              tunnel: w649 -> [w1121]
              tunnel: w648 -> [w1116]
              tunnel: w647 -> [w1115]
              tunnel: [w1106] -> w556
              tunnel: [w1121] -> w555
              tunnel: [w1116] -> w554
              tunnel: [w1115] -> w553
              tunnel: w596 -> [w1119]
              tunnel: [w1119] -> w552
              tunnel: w584 -> [w1118]
              tunnel: [w1118] -> w551
              tunnel: [w1117] -> w550
              tunnel: w579 -> [w1114]
              tunnel: w578 -> [w1099]
              tunnel: w577 -> [w1100]
              tunnel: [w1111] -> w549
              tunnel: w567 -> [w1113]
              tunnel: w566 -> [w1111]
              tunnel: [w1107] -> w548
              tunnel: w559 -> [w1112]
              tunnel: [w1097] -> w547
              tunnel: w546 -> [w1097]
              tunnel: [w1099] -> w545
              tunnel: w521 -> [w1098]
              tunnel: [w1098] -> w520
              tunnel: [w1100] -> w518
              tunnel: w509 -> [w1110]
              tunnel: [w1109] -> w494
              tunnel: w493 -> [w1109]
              tunnel: w479 -> [w1105]
              tunnel: [w1105] -> w478
              tunnel: w474 -> [w1104]
              tunnel: [w1104] -> w473
              tunnel: w468 -> [w1103]
              tunnel: [w1103] -> w467
              tunnel: w463 -> [w1102]
              tunnel: [w1101] -> w462
              tunnel: w459 -> [w1095]
              tunnel: [w1095] -> w458
              tunnel: w453 -> [w1094]
              tunnel: [w1094] -> w452
              tunnel: w449 -> [w1093]
              tunnel: [w1093] -> w448
              tunnel: [w1092] -> w442
              tunnel: w557 -> [w1244]
              tunnel: [w1244] -> w542
              tunnel: w556 -> [w1226]
              tunnel: [w1226] -> w540
              tunnel: w555 -> [w1243]
              tunnel: [w1243] -> w538
              tunnel: w554 -> [w1242]
              tunnel: [w1242] -> w536
              tunnel: w553 -> [w1241]
              tunnel: [w1241] -> w534
              tunnel: w552 -> [w1240]
              tunnel: [w1240] -> w532
              tunnel: w551 -> [w1239]
              tunnel: [w1239] -> w530
              tunnel: w550 -> [w1238]
              tunnel: [w1238] -> w528
              tunnel: w549 -> [w1237]
              tunnel: [w1237] -> w526
              tunnel: [w1231] -> w524
              tunnel: w548 -> [w1230]
              tunnel: w547 -> [w1235]
              tunnel: w545 -> [w1234]
              tunnel: w520 -> [w1223]
              tunnel: [w1223] -> w519
              tunnel: w518 -> [w1225]
              tunnel: [w1225] -> w517
              tunnel: [w1232] -> w516
              tunnel: [w1233] -> w495
              tunnel: w494 -> [w1233]
              tunnel: w478 -> [w1229]
              tunnel: [w1229] -> w477
              tunnel: w473 -> [w1228]
              tunnel: [w1228] -> w472
              tunnel: w467 -> [w1227]
              tunnel: [w1227] -> w466
              tunnel: w462 -> [w1224]
              tunnel: w458 -> [w1221]
              tunnel: [w1224] -> w457
              tunnel: [w1221] -> w456
              tunnel: w452 -> [w1220]
              tunnel: [w1220] -> w451
              tunnel: w448 -> [w1219]
              tunnel: [w1219] -> w447
              tunnel: w442 -> [w1218]
              tunnel: [w1218] -> w441
              tunnel: [w1311] -> w544
              tunnel: [w1323] -> w543
              tunnel: w542 -> [w1338]
              tunnel: [w1338] -> w541
              tunnel: w540 -> [w1317]
              tunnel: [w1317] -> w539
              tunnel: w538 -> [w1337]
              tunnel: [w1337] -> w537
              tunnel: w536 -> [w1336]
              tunnel: [w1336] -> w535
              tunnel: w534 -> [w1335]
              tunnel: [w1335] -> w533
              tunnel: w532 -> [w1334]
              tunnel: [w1334] -> w531
              tunnel: w530 -> [w1333]
              tunnel: [w1333] -> w529
              tunnel: w528 -> [w1332]
              tunnel: [w1332] -> w527
              tunnel: w526 -> [w1331]
              tunnel: [w1331] -> w525
              tunnel: w524 -> [w1330]
              tunnel: [w1330] -> w523
              tunnel: [w1314] -> w522
              tunnel: w519 -> [w1328]
              tunnel: w517 -> [w1327]
              tunnel: w516 -> [w1322]
              tunnel: ["DeltaC Target Setting(pF)"] -> w507
              tunnel: [w1325] -> w496
              tunnel: w495 -> [w1325]
              tunnel: w489 -> [w1324]
              tunnel: [w1324] -> w488
              tunnel: w477 -> [w1321]
              tunnel: [w1321] -> w476
              tunnel: w472 -> [w1320]
              tunnel: [w1320] -> w471
              tunnel: w466 -> [w1319]
              tunnel: [w1319] -> w465
              tunnel: w457 -> [w1318]
              tunnel: w456 -> [w1315]
              tunnel: [w1314] -> w454
              tunnel: w451 -> [w1313]
              tunnel: [w1313] -> w450
              tunnel: w447 -> [w1312]
              tunnel: [w1312] -> w446
              tunnel: w441 -> [w1311]
              tunnel: [w1405] -> w646
              tunnel: [w1425] -> w645
              tunnel: w544 -> [w1405]
              tunnel: w543 -> [w1439]
              tunnel: [w1448] -> w644
              tunnel: [w1439] -> w643
              tunnel: [w1461] -> w642
              tunnel: [w1460] -> w641
              tunnel: w541 -> [w1459]
              tunnel: [w1459] -> w640
              tunnel: w539 -> [w1448]
              tunnel: w537 -> [w1458]
              tunnel: [w1458] -> w639
              tunnel: w535 -> [w1454]
              tunnel: [w1454] -> w638
              tunnel: w533 -> [w1453]
              tunnel: [w1453] -> w637
              tunnel: w531 -> [w1449]
              tunnel: [w1449] -> w595
              tunnel: w529 -> [w1457]
              tunnel: [w1457] -> w583
              tunnel: w527 -> [w1456]
              tunnel: [w1455] -> w580
              tunnel: w525 -> [w1451]
              tunnel: w523 -> [w1447]
              tunnel: [w1452] -> w576
              tunnel: [w1450] -> w575
              tunnel: [w1447] -> w570
              tunnel: w522 -> [w1446]
              tunnel: [w1433] -> w565
              tunnel: [w1432] -> w564
              tunnel: [w1431] -> w563
              tunnel: w507 -> [w1445]
              tunnel: [w1430] -> w497
              tunnel: w496 -> [w1430]
              tunnel: [w1429] -> w492
              tunnel: w488 -> [w1428]
              tunnel: w476 -> [w1423]
              tunnel: w471 -> [w1422]
              tunnel: [w1422] -> w470
              tunnel: w465 -> [w1421]
              tunnel: [w1421] -> w464
              tunnel: w454 -> [w1418]
              tunnel: w450 -> [w1417]
              tunnel: w446 -> [w1406]
              tunnel: w646 -> [w1656]
              tunnel: [w1656] -> w636
              tunnel: [w1683] -> w635
              tunnel: [w1697] -> w634
              tunnel: w645 -> [w1696]
              tunnel: w644 -> [w1695]
              tunnel: w643 -> [w1694]
              tunnel: [w1695] -> w633
              tunnel: [w1694] -> w632
              tunnel: w642 -> [w1693]
              tunnel: [w1693] -> w631
              tunnel: w641 -> [w1692]
              tunnel: [w1692] -> w630
              tunnel: w640 -> [w1691]
              tunnel: [w1691] -> w629
              tunnel: w639 -> [w1690]
              tunnel: [w1690] -> w628
              tunnel: w638 -> [w1689]
              tunnel: [w1689] -> w627
              tunnel: w637 -> [w1688]
              tunnel: [w1688] -> w626
              tunnel: w654 -> [w1687]
              tunnel: [w1685] -> w625
              tunnel: [w1665] -> w624
              tunnel: [w1666] -> w623
              tunnel: [w1664] -> w622
              tunnel: w595 -> [w1681]
              tunnel: [w1681] -> w594
              tunnel: w583 -> [w1680]
              tunnel: [w1680] -> w582
              tunnel: w580 -> [w1697]
              tunnel: w576 -> [w1678]
              tunnel: w575 -> [w1679]
              tunnel: [w1679] -> w574
              tunnel: [w1678] -> w572
              tunnel: w570 -> [w1677]
              tunnel: [w1677] -> w569
              tunnel: w565 -> [w1663]
              tunnel: w564 -> [w1662]
              tunnel: w563 -> [w1661]
              tunnel: [w1658] -> w562
              tunnel: [w1663] -> w515
              tunnel: [w1662] -> w513
              tunnel: [w1661] -> w511
              tunnel: [w1660] -> w498
              tunnel: w497 -> [w1660]
              tunnel: w492 -> [w1659]
              tunnel: [w1659] -> w491
              tunnel: w470 -> [w1658]
              tunnel: w464 -> [w1657]
              tunnel: w636 -> [w1805]
              tunnel: [w1805] -> w621
              tunnel: w635 -> [w1829]
              tunnel: [w1828] -> w620
              tunnel: w670 -> [w1830]
              tunnel: w669 -> [w1827]
              tunnel: w668 -> [w1826]
              tunnel: w667 -> [w1825]
              tunnel: [w1824] -> w619
              tunnel: w634 -> [w1818]
              tunnel: [w1818] -> w618
              tunnel: w633 -> [w1823]
              tunnel: w632 -> [w1822]
              tunnel: [w1823] -> w617
              tunnel: [w1822] -> w616
              tunnel: [w1813] -> w615
              tunnel: w631 -> [w1821]
              tunnel: [w1821] -> w614
              tunnel: w630 -> [w1820]
              tunnel: [w1820] -> w613
              tunnel: w629 -> [w1817]
              tunnel: [w1819] -> w612
              tunnel: w487 -> [w1816]
              tunnel: [w1815] -> w611
              tunnel: [w1803] -> w610
              tunnel: w628 -> [w1814]
              tunnel: w627 -> [w1812]
              tunnel: w626 -> [w1811]
              tunnel: "File Name" -> [w1810]
              tunnel: w625 -> [w1809]
              tunnel: [w1809] -> w609
              tunnel: w624 -> [w1808]
              tunnel: [w1808] -> w608
              tunnel: [w1807] -> w607
              tunnel: w623 -> [w1807]
              tunnel: w622 -> [w1806]
              tunnel: [w1806] -> w606
              tunnel: [w1801] -> w597
              tunnel: w594 -> [w1802]
              tunnel: [w1802] -> w592
              tunnel: w589 -> [w1800]
              tunnel: w582 -> [w1799]
              tunnel: [w1799] -> w581
              tunnel: w574 -> [w1798]
              tunnel: [w1798] -> w573
              tunnel: w572 -> [w1797]
              tunnel: [w1797] -> w571
              tunnel: w569 -> [w1796]
              tunnel: [w1796] -> w568
              tunnel: w562 -> [w1795]
              tunnel: w515 -> [w1794]
              tunnel: [w1794] -> w514
              tunnel: w513 -> [w1793]
              tunnel: [w1793] -> w512
              tunnel: w511 -> [w1792]
              tunnel: [w1792] -> w510
              tunnel: w501 -> [w1791]
              tunnel: [w1791] -> w500
              tunnel: [w1790] -> w499
              tunnel: w498 -> [w1790]
              tunnel: w491 -> [w1789]
              tunnel: [w1789] -> w490
              tunnel: ["Freq(Hz)"] -> w461
              tunnel: ["Board#"] -> w460
              tunnel: w621 -> [w1851]
              tunnel: w620 -> [w1902]
              tunnel: w670 -> [w1866]
              tunnel: w666 -> [w1897]
              tunnel: w665 -> [w1900]
              tunnel: w664 -> [w1896]
              tunnel: w663 -> [w1899]
              tunnel: w662 -> [w1895]
              tunnel: w619 -> [w1898]
              tunnel: [w1851] -> w602
              tunnel: [w1901] -> w603
              tunnel: w618 -> [w1894]
              tunnel: [w1894] -> w604
              tunnel: w617 -> [w1893]
              tunnel: w616 -> [w1878]
              tunnel: w615 -> [w1892]
              tunnel: w614 -> [w1891]
              tunnel: w613 -> [w1880]
              tunnel: [w1888] -> w605
              tunnel: w612 -> [w1890]
              tunnel: w611 -> [w1889]
              tunnel: w610 -> [w1888]
              tunnel: "File Name" -> [w1859]
              tunnel: w609 -> [w1887]
              tunnel: [w1887] -> w601
              tunnel: w608 -> [w1886]
              tunnel: w607 -> [w1885]
              tunnel: w606 -> [w1884]
              tunnel: [w1883] -> w598
              tunnel: w597 -> [w1883]
              tunnel: [w1862] -> w593
              tunnel: w592 -> [w1862]
              tunnel: w581 -> [w1882]
              tunnel: w573 -> [w1881]
              tunnel: w571 -> [w1879]
              tunnel: w568 -> [w1877]
              tunnel: w514 -> [w1876]
              tunnel: w512 -> [w1875]
              tunnel: w510 -> [w1874]
              tunnel: w508 -> [w1873]
              tunnel: w438 -> [w1872]
              tunnel: w503 -> [w1871]
              tunnel: w506 -> [w1870]
              tunnel: w500 -> [w1869]
              tunnel: w499 -> [w1868]
              tunnel: w490 -> [w1867]
              tunnel: [w1864] -> w486
              tunnel: [w1855] -> w482
              tunnel: w461 -> [w1854]
              tunnel: w460 -> [w1852]
              tunnel: [w1952] -> w660
              tunnel: [w1953] -> w661
              tunnel: [w1954] -> w561
              tunnel: w605 -> [w1945]
              tunnel: w604 -> [w1953]
              tunnel: w603 -> [w1941]
              tunnel: w602 -> [w1954]
              tunnel: w601 -> [w1947]
              tunnel: [w1947] -> w653
              tunnel: [w1944] -> w590
              tunnel: w598 -> [w1944]
              tunnel: w593 -> [w1946]
              tunnel: [w1946] -> w591
              tunnel: [w1945] -> w588
              tunnel: [w1943] -> w587
              tunnel: [w1940] -> w483
              tunnel: w486 -> [w1939]
              tunnel: w482 -> [w1937]
              frame #0 {
                w745 = FALSE ("Log (T)")
                n137 = call "WSVCAP SHL Host TL RFFE Write - Multiple DUTs - Common Data.vi"("Data Out"=w766, "error in"=w771, "Log (T)"=FALSE) -> ("error out"=w752:errorcluster)  [unwired: 12 in]
                n138 = Index Array(array=w781, index (row)=w775, index (col)=0 ("disabled index (col)")) -> (element=w774:dbl)
                n139 = for {
                  tunnel: string[] ["0760", "0767", "0768"] -> [w850] mode=indexing
                  tunnel: [w846] -> w756 mode=indexing
                  tunnel: w752 -> [w844]
                  tunnel: [w843] -> w753
                  i -> [w849]
                  n140 = call "Delay.vi"("milliseconds to wait"=u32 10, "error in (no error)"=w844) -> ("error out"=w851:errorcluster)  [unwired: 9 in]
                  n141 = call "WSVCAP SHL Host TL RFFE Read - Multiple DUTs - Common Data.vi"("Data Out"=w850, "error in"=w851, "Log (T)"=FALSE) -> ("RFFE Data In"=w848:string[], "error out"=w843:errorcluster)  [unwired: 11 in]
                  n142 = Index Array(array=w848, index=w849) -> (element=w845:string)
                  n143 = String Subset(string=w845, offset (0)=0) -> (substring=w846:string)  [unwired: 1 in]
                }
                "RB Reg for HD/Cycle" <- w756
                n144 = local read "IDD Brd(uA)"() -> (w765:string)
                n145 = call "Delay.vi"("milliseconds to wait"=u32 100, "error in (no error)"=w753) -> ("error out"=w761:errorcluster)  [unwired: 9 in]
                n146 = call "Ke2000 Single Reading.vi"("error in (no error)"=w761, "VISA resource name"=w758) -> ("error out"=w763:errorcluster, "VISA resource name out"=w733:refnum<visa-resource-name>, "uA"=w764:string)  [unwired: 5 in, 2 out]
                n147 = call "Substration.vi"("error in (no error)"=w763, "Input2"=w765, "Input1"=w764) -> ("error out"=w760:errorcluster, "In1 - In2"=→"IDD_HD/CYC (uA)":string)  [unwired: 7 in]
                n148 = case shown="True" w773 {
                  tunnel: [w882 w987] -> w783
                  tunnel: [w883 w972] -> w719
                  tunnel: [w881 w988] -> w780
                  tunnel: w760 -> [w877 w976]
                  tunnel: w776 -> [_ w978]
                  tunnel: w774 -> [w874 w973]
                  tunnel: [w879 w974] -> w772
                  tunnel: w754 -> [w866 w970]
                  tunnel: w769 -> [w876 _]
                  tunnel: ["% Duty Cycle" "100" ("Data Out")] -> w755
                  tunnel: w751 -> [w864 _]
                  tunnel: w734 -> [w863 w965]
                  tunnel: w723 -> [w860 _]
                  tunnel: w722 -> [w859 _]
                  frame False {
                    # "Cycles in 1s"
                    n149 = case shown="True" w863 {
                      tunnel: w877 -> [w889 w895]
                      tunnel: w874 -> [w888 w894]
                      tunnel: [w887 w895] -> w873
                      tunnel: w866 -> [w886 _]
                      tunnel: [w885 w894] -> w872
                      tunnel: [u64 1000 ("y") u64 1 ("y")] -> w867
                      frame False {
                        n150 = case shown="8, Default" w886 {
                          tunnel: w888 -> [w891 _]
                          tunnel: [w891 "Cycle RP"] -> w885
                          tunnel: [w890 w892] -> w887
                          tunnel: w889 -> [w890 w892]
                          frame 0..7 {
                          }
                          frame 8, Default {
                          }
                        }
                      }
                      frame True {
                        # "Read real number\nfrom lookup table"
                      }
                    }
                    n151 = call "WSVCAP SHL Host TL RFFE Configure.vi"("RFFE Slave Address"=w876, "Clock Rate (Hz)"="SPI Clock Rate (Hz)", "error in"=w873) -> ("Actual Rate (Hz)"=→"AR Cycling(Hz)":dbl, "error out"=w862:errorcluster)  [unwired: 11 in]
                    n152 = Array Max & Min(array=w859) -> (max value=w870:dbl)  [unwired: 3 out]
                    n153 = Divide(x=1.0, y=w870) -> (x/y=w869:dbl)
                    n154 = To Unsigned Quad Integer(1:w869) -> (0:w868:u64)
                    n155 = Not(x=w864) -> (.not. x?=w865:bool)
                    n156 = case shown="True" w865 {
                      tunnel: [w898 w920] -> w883
                      tunnel: [w901 w919] -> w882
                      tunnel: [u64 1 w918] -> w881
                      tunnel: w862 -> [w899 w917]
                      tunnel: w872 -> [_ w916]
                      tunnel: w859 -> [_ w914]
                      tunnel: w868 -> [_ w913]
                      tunnel: w867 -> [_ w912]
                      tunnel: w866 -> [w897 _]
                      tunnel: w860 -> [_ w911]
                      frame False {
                        n157 = case shown="1, Default" w897 {
                          tunnel: w899 -> [w902 w904]
                          tunnel: [w902 w903] -> w898
                          frame 0 {
                          }
                          frame 1, Default {
                            n158 = flat-sequence {
                              tunnel: "Repeat Meas(s)" -> [w910]
                              tunnel: w904 -> [w907]
                              tunnel: [w907] -> w903
                              frame #0 {
                                n159 = Multiply(x=w910, y=u32 1000) -> (x*y=w909:u32)
                                n160 = Wait (ms)(milliseconds to wait=w909) -> ()  [unwired: 1 out]
                                n161 = local write "STATUS"("Verify Sockets waiting times..." ("STATUS")) -> ()
                              }
                            }
                          }
                        }
                        n162 = local read "stop During HD/Cycles"() -> (w901:bool)
                      }
                      frame True {
                        n163 = while {
                          tunnel: w916 -> [w940]
                          tunnel: [w927] -> w920
                          tunnel: [w932] -> w919
                          tunnel: w917 -> [w938]
                          tunnel: [w926] -> w918
                          tunnel: w911 -> [w937]
                          tunnel: w914 -> [w936]
                          tunnel: w913 -> [w923]
                          tunnel: w912 -> [w921]
                          i -> [w935]
                          stop <- w931 stop-if-true
                          # "At least 1 second before target"
                          # "Remaining Cycles"
                          # "Target Cycles"
                          # "Cycles in 1s"
                          n164 = To Unsigned Quad Integer(1:w940) -> (0:w939:u64)
                          n165 = case shown="0" w935 {
                            tunnel: [w948 w950] -> w929
                            tunnel: w938 -> [w949 w950]
                            tunnel: w937 -> [w947 _]
                            tunnel: w936 -> [w946 _]
                            frame 0 {
                              n166 = call "WSVCAP SHL Host TL RFFE Write Cycle - Multiple DUTs - Common Data.vi"("Data Out (Cycle Commands)"=w947, "Post Command Delay"=w946, "error in"=w949, "Log (T)"=FALSE) -> ("error out"=w948:errorcluster)  [unwired: 11 in]
                            }
                            frame 1, Default {
                            }
                          }
                          n167 = Multiply(x=w939, y=w921) -> (x*y=w926:u64)
                          n168 = call "WSVCAP SHL Host TL SPI_RFFE Query Cycle Count.vi"("error in"=w929) -> ("Cycle Count"=w925:u64, "error out"=w934:errorcluster)  [unwired: 13 in]
                          "Cycle Count" <- w925
                          n169 = Subtract(x=w926, y=w925) -> (x-y=w924:u64)
                          n170 = Greater Or Equal?(x=w925, y=w926) -> (x >= y?=w933:bool)
                          n171 = local read "stop During HD/Cycles"() -> (w932:bool)
                          n172 = Greater?(x=w924, y=w923) -> (0:w922:bool)
                          n173 = case shown="True" w933 {
                            tunnel: [w952 w955] -> w928
                            tunnel: w934 -> [w952 w954]
                            tunnel: [FALSE TRUE] -> w930
                            frame False {
                            }
                            frame True {
                              n174 = call "WSVCAP SHL Host TL SPI Stop Write Cycle.vi"("error in"=w954) -> ("error out"=w955:errorcluster)  [unwired: 14 in]
                            }
                          }
                          n175 = Or(x=w930, y=w932) -> (x .or. y?=w931:bool)
                          n176 = case shown="True" w922 {
                            tunnel: w928 -> [w941 w944]
                            tunnel: [w941 w943] -> w927
                            frame False {
                            }
                            frame True {
                              n177 = call "MISC Wait with Data Flow.vi"("Error In (no error)"=w944, "Wait Time (500ms)"=u32 50) -> ("Error Out"=w943:errorcluster)  [unwired: 7 in, 2 out]
                            }
                          }
                        }
                        n178 = local write "STATUS"("Parts are Cycling...." ("STATUS")) -> ()
                      }
                    }
                    n179 = local read "HD/CYC Temp"() -> (w878:i32)
                    n180 = Number To Engineering String(4:w878) -> (0:w879:string)  [unwired: 3 in]
                  }
                  frame True {
                    n181 = case shown="False" w965 {
                      tunnel: w978 -> [w1005 _]
                      tunnel: [w1004 w1017] -> w977
                      tunnel: w976 -> [w1003 w1018]
                      tunnel: [w1002 w1018] -> w975
                      tunnel: w973 -> [w1001 w1017]
                      tunnel: w970 -> [w1000 _]
                      frame False {
                        n182 = case shown="1, Default" w1005 {
                          tunnel: [w1008 w1015] -> w1004
                          tunnel: w1003 -> [w1010 w1016]
                          tunnel: [w1009 w1016] -> w1002
                          tunnel: w1001 -> [w1007 _]
                          tunnel: w1000 -> [w1006 _]
                          frame 0 {
                            n183 = case shown="15, Default" w1006 {
                              tunnel: [w1011 "HD RP"] -> w1008
                              tunnel: w1010 -> [w1012 w1013]
                              tunnel: [w1012 w1013] -> w1009
                              tunnel: w1007 -> [w1011 _]
                              frame 0..14 {
                              }
                              frame 15, Default {
                              }
                            }
                          }
                          frame 1, Default {
                            n184 = local read "HD RP"() -> (w1015:dbl)
                          }
                        }
                      }
                      frame True {
                      }
                    }
                    n185 = call "WSVCAP SHL Host TL RFFE Write - Multiple DUTs - Common Data.vi"("Data Out"="Cmd To HD", "error in"=w975, "Log (T)"=FALSE) -> ("error out"=w961:errorcluster)  [unwired: 12 in]
                    n186 = local read "No of HD/Cycle\nCompleted"() -> (w979:u64)
                    n187 = call "Delay.vi"("milliseconds to wait"=u32 50, "error in (no error)"=w961) -> ("error out"=w958:errorcluster)  [unwired: 9 in]
                    n188 = for {
                      tunnel: string[] ["0761", "0762", "0763"] -> [w999] mode=indexing
                      tunnel: [w995] -> w957 mode=indexing
                      shift-right: [w992] -> w983
                      shift-left: w958 -> [w998]
                      i -> [w997]
                      n189 = call "WSVCAP SHL Host TL RFFE Read - Multiple DUTs - Common Data.vi"("Data Out"=w999, "error in"=w998, "Log (T)"=FALSE) -> ("RFFE Data In"=w994:string[], "error out"=w991:errorcluster)  [unwired: 11 in]
                      n190 = Index Array(array=w994, index=w997) -> (element=w993:string)
                      n191 = call "Delay.vi"("milliseconds to wait"=u32 10, "error in (no error)"=w991) -> ("error out"=w992:errorcluster)  [unwired: 9 in]
                      n192 = String Subset(string=w993, offset (0)=0) -> (substring=w995:string)  [unwired: 1 in]
                    }
                    "RB Reg for HD" <- w957
                    n193 = Greater?(x="HD_DC (Min)", y=w979) -> (0:w980:bool)
                    n194 = case shown="True" w980 {
                      tunnel: [_ w1029] -> w985
                      tunnel: [w1020 w1028] -> w984
                      tunnel: w983 -> [w1020 w1027]
                      tunnel: w977 -> [w1019 w1026]
                      tunnel: [w1019 w1026] -> w982
                      frame False {
                      }
                      frame True {
                        n195 = Multiply(x=1000.0, y=w1026) -> (x*y=w1024:dbl)
                        n196 = Multiply(x=60.0, y=w1024) -> (x*y=w1022:dbl)
                        n197 = local write "STATUS"("Parts are Holding Down..." ("STATUS")) -> ()
                        n198 = event shown="[0] Timeout" {
                          selector: _ -> [_ _]
                          dyn-events: _ -> [_ _]
                          timeout: w1022 -> [_ _]
                          tunnel: ["stop During HD/Cycles" TRUE ("stop During HD/Cycles")] -> w1029
                          tunnel: w1027 -> [w1030 w1032]
                          tunnel: [w1030 w1032] -> w1028
                          event Timeout {
                            n199 = event-data() -> ()  [unwired: 1 in, 2 out]
                          }
                          event "stop During HD/Cycles": Value Change {
                            n200 = event-data() -> ()  [unwired: 1 in, 2 out]
                          }
                        }
                      }
                    }
                    n201 = Greater Or Equal?(x=w979, y="HD_DC (Min)") -> (x >= y?=w986:bool)
                    n202 = To Unsigned Quad Integer(1:w977) -> (0:w988:u64)
                    n203 = Add(x="Time All OFF (s)", y="Time All ON (s)") -> (x+y=w967:u32)
                    n204 = To Double Precision Float(number=w967) -> (double precision float=w966:dbl)
                    n205 = Divide(x=w966, y=60.0) -> (x/y=w968:dbl)
                    n206 = case shown="False" w986 {
                      tunnel: [w1036 w1052] -> w987
                      tunnel: [w1037 w1044] -> w972
                      tunnel: w984 -> [w1037 w1051]
                      tunnel: w985 -> [w1036 w1050]
                      tunnel: w982 -> [_ w1049]
                      tunnel: [w1035 w1047] -> w974
                      tunnel: w968 -> [_ w1041]
                      tunnel: "Time All OFF (s)" -> [_ w1039]
                      tunnel: "Time All ON (s)" -> [_ w1038]
                      frame False {
                        n207 = Number To Engineering String(4:"HD/CYC Temp") -> (0:w1035:string)  [unwired: 3 in]
                      }
                      frame True {
                        n208 = Divide(x=w1049, y=w1041) -> (x/y=w1048:dbl)
                        n209 = call "WSVCAP SHL Host TL RFFE Write - Multiple DUTs - Common Data.vi"("Data Out"="070201000000", "error in"=w1051, "Log (T)"=FALSE) -> ("error out"=w1054:errorcluster)  [unwired: 12 in]
                        n210 = Round To Nearest(number=w1048) -> (nearest integer value=w1043:dbl)
                        n211 = call "Delay.vi"("milliseconds to wait"=u32 50, "error in (no error)"=w1054) -> ("error out"=w1045:errorcluster)  [unwired: 9 in]
                        n212 = To Long Integer(number=w1043) -> (32bit integer=w1042:i32)
                        "No LPs to RP" <- w1042
                        n213 = for {
                          N: w1042 -> [_]
                          tunnel: w1050 -> [w1072]
                          tunnel: [w1071] -> w1052
                          tunnel: w1045 -> [w1061]
                          tunnel: [w1060] -> w1044
                          tunnel: w1039 -> [w1058]
                          tunnel: w1038 -> [w1056]
                          i -> [w1070]
                          stop <- w1071 stop-if-true
                          w1059 = FALSE ("Log (T)")
                          w1057 = u32 1 ("milliseconds to wait")
                          n214 = Increment(x=w1070) -> (x+1=→"LPs Count":i32)
                          n215 = call "WSVCAP SHL Host TL RFFE Write - Multiple DUTs - Common Data.vi"("Data Out"="074776", "error in"=w1061, "Log (T)"=w1059) -> ("error out"=w1078:errorcluster)  [unwired: 12 in]
                          n216 = call "Delay.vi"("milliseconds to wait"=w1057, "error in (no error)"=w1078) -> ("error out"=w1077:errorcluster)  [unwired: 9 in]
                          n217 = local read "CP to HD/Cycle"() -> (w1063:i32)
                          n218 = call "WSVCAP SHL Host TL RFFE Write - Multiple DUTs - Common Data.vi"("Data Out"="070201000000", "error in"=w1064) -> ("error out"=w1074:errorcluster)  [unwired: 13 in]
                          n219 = call "WSVCAP SHL Host TL RFFE Write - Multiple DUTs - Common Data.vi"("Data Out"="0702013B3B3B", "error in"=w1077, "Log (T)"=w1059) -> ("error out"=w1067:errorcluster)  [unwired: 12 in]
                          n220 = call "Delay.vi"("milliseconds to wait"=w1057, "error in (no error)"=w1067) -> ("error out"=w1066:errorcluster)  [unwired: 9 in]
                          n221 = flat-sequence {
                            tunnel: w1074 -> [w1085]
                            tunnel: [w1083] -> w1060
                            tunnel: w1058 -> [w1080]
                            frame #0 {
                              n222 = local write "STATUS"("Now HD OFF Time..." ("STATUS")) -> ()
                              n223 = Multiply(x=w1080, y=u32 1000) -> (x*y=w1082:u32)
                              n224 = call "Delay.vi"("milliseconds to wait"=w1082, "error in (no error)"=w1085) -> ("error out"=w1083:errorcluster)  [unwired: 9 in]
                            }
                          }
                          n225 = Index Array(array=string[] ["07476F", "074776", "074765", "074769", "07477B"], index=w1063) -> (element=w1068:string)
                          n226 = call "WSVCAP SHL Host TL RFFE Write - Multiple DUTs - Common Data.vi"("Data Out"=w1068, "error in"=w1066, "Log (T)"=w1059) -> ("error out"=w1065:errorcluster)  [unwired: 12 in]
                          n227 = flat-sequence {
                            tunnel: [w1090] -> w1064
                            tunnel: w1065 -> [w1087]
                            tunnel: w1056 -> [w1086]
                            frame #0 {
                              n228 = local write "STATUS"("Now HD ON Time..." ("STATUS")) -> ()
                              n229 = Multiply(x=w1086, y=u32 1000) -> (x*y=w1089:u32)
                              n230 = call "Delay.vi"("milliseconds to wait"=w1089, "error in (no error)"=w1087) -> ("error out"=w1090:errorcluster)  [unwired: 9 in]
                            }
                          }
                          n231 = Unbundle By Name(w1060) -> ("status"=w1073:bool)
                          n232 = Or(x=w1073, y=w1072) -> (x .or. y?=w1071:bool)
                        }
                        n233 = Number To Engineering String(4:"DC_Temp") -> (0:w1047:string)  [unwired: 3 in]
                      }
                    }
                  }
                }
                n234 = case shown="0, Default" "CP to Meas" {
                  selector: "CP to Meas" -> [w787 w792 w797 w802 w807 w812 w817 w822 w826]
                  tunnel: string[] ["07476F", "074776", "074765", "074769", "07477B", "07477C", "07477D", "074779", "07476B"] -> [w788 w793 w798 w803 w808 w813 w818 w823 w828]
                  tunnel: [w786 w791 w796 w801 w806 w811 w816 w821 w827] -> w717
                  tunnel: ["35.0" ("Data Out") "27.5" ("Data Out") "30.5" ("Data Out") "44.0" ("Data Out") "50.0" ("Data Out") "55.0" ("Data Out") "42.5" ("Data Out") "32.0" ("Data Out") "40.25" ("Data Out")] -> w721
                  tunnel: [w784 w789 w794 w799 w804 w809 w814 w819 w824] -> w720
                  tunnel: w719 -> [w784 w789 w794 w799 w804 w809 w814 w819 w824]
                  frame 0, Default {
                    n235 = Index Array(array=w788, index=w787) -> (element=w786:string)
                  }
                  frame 2 {
                    n236 = Index Array(array=w793, index=w792) -> (element=w791:string)
                  }
                  frame 3 {
                    n237 = Index Array(array=w798, index=w797) -> (element=w796:string)
                  }
                  frame 4 {
                    n238 = Index Array(array=w803, index=w802) -> (element=w801:string)
                  }
                  frame 5 {
                    n239 = Index Array(array=w808, index=w807) -> (element=w806:string)
                  }
                  frame 6 {
                    n240 = Index Array(array=w813, index=w812) -> (element=w811:string)
                  }
                  frame 7 {
                    n241 = Index Array(array=w818, index=w817) -> (element=w816:string)
                  }
                  frame 8 {
                    n242 = Index Array(array=w823, index=w822) -> (element=w821:string)
                  }
                  frame 1 {
                    n243 = Index Array(array=w828, index=w826) -> (element=w827:string)
                  }
                }
                n244 = call "WSVCAP SHL Host TL RFFE Write - Multiple DUTs - Common Data.vi"("Data Out"=w717, "error in"=w720, "Log (T)"=w745) -> ("error out"=w767:errorcluster)  [unwired: 12 in]
                n245 = flat-sequence {
                  tunnel: w747 -> [w853]
                  tunnel: [w853] -> w743
                  frame #0 {
                    w855 = "0" ("NOM IDD OFF(uA)")
                    w856 = string[] []
                    w857 = string[][] []
                    n246 = To Long Integer(number=0.0 ("No of Loops to RP")) -> (32bit integer=w854:i32)
                    n247 = local write "NOM IDD ON (uA)"(w855) -> ()
                    n248 = local write "NOM IDD OFF(uA)"(w855) -> ()
                    n249 = local write "LPs Count"(w854) -> ()
                    n250 = local write "No LPs to RP"(w854) -> ()
                    n251 = local write "Total Delta C1(pF)"(w856) -> ()
                    n252 = local write "Total Delta C2(pF)"(w856) -> ()
                    n253 = local write "Total Delta C3(pF)"(w856) -> ()
                    n254 = local write "Current EFuse Read back"(w856) -> ()
                    n255 = local write "RB Reg for HD"(w856) -> ()
                    n256 = local write "RB Reg for HD/Cycle"(w856) -> ()
                    n257 = local write "CAP_C3"(w857) -> ()
                    n258 = local write "CAP_C2"(w857) -> ()
                    n259 = local write "CAP_C1"(w857) -> ()
                    n260 = local write "VSA_V3"(w857) -> ()
                    n261 = local write "VSA_V1"(w857) -> ()
                    n262 = local write "VSA_V2"(w857) -> ()
                    n263 = local write "VPI C1"(w857) -> ()
                    n264 = local write "VPI C2"(w857) -> ()
                    n265 = local write "VPI C3"(w857) -> ()
                    n266 = local write "% Delta C"(w857) -> ()
                  }
                }
                n267 = call "Delay.vi"("milliseconds to wait"=u32 50, "error in (no error)"=w767) -> ("error out"=w726:errorcluster)  [unwired: 9 in]
                n268 = for {
                  tunnel: [w841] -> w778
                  tunnel: [w840] -> w747
                  tunnel: w745 -> [w839]
                  tunnel: w733 -> [w838]
                  tunnel: w726 -> [w834]
                  tunnel: string[] ["0702013B3B3B", "070201000000"] -> [w830] mode=indexing
                  tunnel: [w829] -> w729 mode=indexing
                  n269 = call "WSVCAP SHL Host TL RFFE Write - Multiple DUTs - Common Data.vi"("Data Out"=w830, "error in"=w834, "Log (T)"=w839) -> ("error out"=w835:errorcluster)  [unwired: 12 in]
                  n270 = local read "IDD Brd(uA)"() -> (w831:string)
                  n271 = call "Delay.vi"("milliseconds to wait"=u32 100, "error in (no error)"=w835) -> ("error out"=w836:errorcluster)  [unwired: 9 in]
                  n272 = call "Ke2000 Single Reading.vi"("error in (no error)"=w836, "VISA resource name"=w838) -> ("error out"=w833:errorcluster, "VISA resource name out"=w841:refnum<visa-resource-name>, "uA"=w832:string)  [unwired: 5 in, 2 out]
                  n273 = call "Substration.vi"("error in (no error)"=w833, "Input2"=w831, "Input1"=w832) -> ("error out"=w840:errorcluster, "In1 - In2"=w829:string)  [unwired: 7 in]
                }
                n274 = Index Array(array=w729, index=1) -> (element=w728:string)
                n275 = Index Array(array=w729, index=0) -> (element=w731:string)
                n276 = local read "Clock Rate (Hz)"() -> (w768:dbl)
                n277 = call "Multi Dut Cmd_Header Setting.vi"("WS1050/51"="WS1050/51", "Cmin/Act"="Cmin/Act", "Test Seq"="Test Sequences", "error in (no error)"=w743) -> ("Name 1"=w741:string[], "Name 2"=w740:string[], "Name Header"=w738:string[], "Name 3"=w739:string[], "Cmd 3"=w735:string[], "Cmd 1"=w737:string[], "Cmd 2"=w736:string[], "error out"=w744:errorcluster)  [unwired: 2 in, 2 out]
              }
              frame #1 {
                w1101 = FALSE ("Log (T)")
                n278 = call "WSVCAP SHL Host TL RFFE Configure.vi"("RFFE Slave Address"=w1112, "Clock Rate (Hz)"=w1110, "error in"=w1102) -> ("Actual Rate (Hz)"=w1120:dbl, "error out"=w1108:errorcluster)  [unwired: 11 in]
                n279 = local write "AR  Measurent(Hz)"(w1120) -> ()
                n280 = Array Size(array=w1113) -> (size(s)=w1123:i32)
                n281 = case shown="False" w1092 {
                  tunnel: w1123 -> [w1131 _]
                  tunnel: w1114 -> [w1130 _]
                  tunnel: w1113 -> [w1129 _]
                  tunnel: w1108 -> [w1128 w1217]
                  tunnel: [w1127 w1217] -> w1107
                  tunnel: w1101 -> [w1126 _]
                  tunnel: [w1125 string[][] []] -> w1096
                  tunnel: w1095 -> [w1124 _]
                  frame False {
                    n282 = case shown="2" w1124 {
                      tunnel: w1131 -> [w1138 w1166 w1194]
                      tunnel: w1130 -> [w1137 w1165 w1193]
                      tunnel: w1129 -> [w1136 w1164 w1192]
                      tunnel: w1128 -> [w1135 w1163 w1191]
                      tunnel: [w1134 w1162 w1190] -> w1127
                      tunnel: w1126 -> [w1133 w1161 w1189]
                      tunnel: [w1132 w1160 w1188] -> w1125
                      frame 0, Default {
                        n283 = for {
                          N: w1138 -> [_]
                          tunnel: w1137 -> [w1155]
                          tunnel: [w1151] -> w1132 mode=indexing
                          tunnel: w1136 -> [w1153]
                          tunnel: w1135 -> [w1141]
                          tunnel: [w1143] -> w1134
                          tunnel: w1133 -> [w1142]
                          i -> [w1150]
                          stop <- w1139 stop-if-true
                          n284 = Index Array(array=w1155, index=w1150) -> (element=w1154:string)
                          n285 = Index Array(array=w1153, index=w1150) -> (element=w1152:string)
                          n286 = local write "STATUS"(w1152) -> ()
                          n287 = call "WSVCAP SHL Host TL RFFE Write - Multiple DUTs - Common Data.vi"("Data Out"=w1154, "error in"=w1141, "Log (T)"=FALSE) -> ("error out"=w1145:errorcluster)  [unwired: 12 in]
                          n288 = call "Delay.vi"("milliseconds to wait"=u32 10, "error in (no error)"=w1145) -> ("error out"=w1149:errorcluster)  [unwired: 9 in]
                          n289 = call "WS1050 AD7747 READ 36 DUT.vi"("error in"=w1149, "Log (T)"=w1142, "DUT Mask Mode (All)"=WSVCAP_SHL_I2C_DUT_Mask_Mode_Enum."C1") -> ("error out"=w1147:errorcluster, "AD7747 Values"=w1148:string[][])  [unwired: 7 in]
                          n290 = for {
                            tunnel: w1148 -> [w1158] mode=indexing
                            tunnel: w1147 -> [w1159]
                            tunnel: [w1159] -> w1143
                            tunnel: [w1156] -> w1151 mode=indexing
                            n291 = Index Array(array=w1158, index=1) -> (element=w1156:string)
                          }
                          n292 = Unbundle By Name(w1143) -> ("status"=w1139:bool)
                        }
                      }
                      frame 1 {
                        n293 = for {
                          N: w1166 -> [_]
                          tunnel: w1165 -> [w1183]
                          tunnel: [w1179] -> w1160 mode=indexing
                          tunnel: w1164 -> [w1181]
                          tunnel: w1163 -> [w1169]
                          tunnel: [w1171] -> w1162
                          tunnel: w1161 -> [w1170]
                          i -> [w1178]
                          stop <- w1167 stop-if-true
                          n294 = Index Array(array=w1183, index=w1178) -> (element=w1182:string)
                          n295 = Index Array(array=w1181, index=w1178) -> (element=w1180:string)
                          n296 = local write "STATUS"(w1180) -> ()
                          n297 = call "WSVCAP SHL Host TL RFFE Write - Multiple DUTs - Common Data.vi"("Data Out"=w1182, "error in"=w1169, "Log (T)"=FALSE) -> ("error out"=w1173:errorcluster)  [unwired: 12 in]
                          n298 = call "Delay.vi"("milliseconds to wait"=u32 10, "error in (no error)"=w1173) -> ("error out"=w1177:errorcluster)  [unwired: 9 in]
                          n299 = call "WS1050 AD7747 READ 36 DUT.vi"("error in"=w1177, "Log (T)"=w1170, "DUT Mask Mode (All)"=WSVCAP_SHL_I2C_DUT_Mask_Mode_Enum."C2") -> ("error out"=w1175:errorcluster, "AD7747 Values"=w1176:string[][])  [unwired: 7 in]
                          n300 = for {
                            tunnel: w1176 -> [w1186] mode=indexing
                            tunnel: w1175 -> [w1187]
                            tunnel: [w1187] -> w1171
                            tunnel: [w1184] -> w1179 mode=indexing
                            n301 = Index Array(array=w1186, index=3) -> (element=w1184:string)
                          }
                          n302 = Unbundle By Name(w1171) -> ("status"=w1167:bool)
                        }
                      }
                      frame 2 {
                        n303 = for {
                          N: w1194 -> [_]
                          tunnel: w1193 -> [w1211]
                          tunnel: [w1207] -> w1188 mode=indexing
                          tunnel: w1192 -> [w1209]
                          tunnel: w1191 -> [w1197]
                          tunnel: [w1199] -> w1190
                          tunnel: w1189 -> [w1198]
                          i -> [w1206]
                          stop <- w1195 stop-if-true
                          n304 = Index Array(array=w1211, index=w1206) -> (element=w1210:string)
                          n305 = Index Array(array=w1209, index=w1206) -> (element=w1208:string)
                          n306 = local write "STATUS"(w1208) -> ()
                          n307 = call "WSVCAP SHL Host TL RFFE Write - Multiple DUTs - Common Data.vi"("Data Out"=w1210, "error in"=w1197, "Log (T)"=FALSE) -> ("error out"=w1201:errorcluster)  [unwired: 12 in]
                          n308 = call "Delay.vi"("milliseconds to wait"=u32 10, "error in (no error)"=w1201) -> ("error out"=w1205:errorcluster)  [unwired: 9 in]
                          n309 = call "WS1050 AD7747 READ 36 DUT.vi"("error in"=w1205, "Log (T)"=w1198, "DUT Mask Mode (All)"=WSVCAP_SHL_I2C_DUT_Mask_Mode_Enum."C3") -> ("error out"=w1203:errorcluster, "AD7747 Values"=w1204:string[][])  [unwired: 7 in]
                          n310 = for {
                            tunnel: w1204 -> [w1214] mode=indexing
                            tunnel: w1203 -> [w1215]
                            tunnel: [w1215] -> w1199
                            tunnel: [w1212] -> w1207 mode=indexing
                            n311 = Index Array(array=w1214, index=5) -> (element=w1212:string)
                          }
                          n312 = Unbundle By Name(w1199) -> ("status"=w1195:bool)
                        }
                      }
                    }
                  }
                  frame True {
                  }
                }
                n313 = Transpose 2D Array(2D array=w1096) -> (transposed array=w1106:string[][])
                "CAP_C1" <- w1106
                "NOM IDD ON (uA)" <- w1116
                "NOM IDD OFF(uA)" <- w1115
              }
              frame #2 {
                n314 = Array Size(array=w1235) -> (size(s)=w1236:i32)
                n315 = case shown="True" w1218 {
                  tunnel: w1236 -> [w1252 _]
                  tunnel: w1235 -> [w1251 _]
                  tunnel: w1234 -> [w1250 _]
                  tunnel: [w1249 w1310] -> w1232
                  tunnel: w1230 -> [w1248 w1310]
                  tunnel: w1224 -> [w1247 _]
                  tunnel: [w1246 string[][] []] -> w1222
                  tunnel: w1221 -> [w1245 _]
                  frame False {
                    n316 = case shown="0, 2, Default" w1245 {
                      tunnel: w1252 -> [w1259 w1287]
                      tunnel: w1251 -> [w1258 w1286]
                      tunnel: w1250 -> [w1257 w1285]
                      tunnel: [w1256 w1284] -> w1249
                      tunnel: w1248 -> [w1255 w1283]
                      tunnel: w1247 -> [w1254 w1282]
                      tunnel: [w1253 w1281] -> w1246
                      frame 0, 2, Default {
                        n317 = for {
                          N: w1259 -> [_]
                          tunnel: w1257 -> [w1276]
                          tunnel: [w1272] -> w1253 mode=indexing
                          tunnel: w1258 -> [w1274]
                          tunnel: w1255 -> [w1262]
                          tunnel: [w1264] -> w1256
                          tunnel: w1254 -> [w1263]
                          i -> [w1271]
                          stop <- w1260 stop-if-true
                          n318 = Index Array(array=w1276, index=w1271) -> (element=w1275:string)
                          n319 = Index Array(array=w1274, index=w1271) -> (element=w1273:string)
                          n320 = call "WSVCAP SHL Host TL RFFE Write - Multiple DUTs - Common Data.vi"("Data Out"=w1275, "error in"=w1262, "Log (T)"=FALSE) -> ("error out"=w1266:errorcluster)  [unwired: 12 in]
                          n321 = local write "STATUS"(w1273) -> ()
                          n322 = call "Delay.vi"("milliseconds to wait"=u32 10, "error in (no error)"=w1266) -> ("error out"=w1270:errorcluster)  [unwired: 9 in]
                          n323 = call "WS1050 AD7747 READ 36 DUT.vi"("error in"=w1270, "Log (T)"=w1263, "DUT Mask Mode (All)"=WSVCAP_SHL_I2C_DUT_Mask_Mode_Enum."C2") -> ("error out"=w1268:errorcluster, "AD7747 Values"=w1269:string[][])  [unwired: 7 in]
                          n324 = for {
                            tunnel: w1269 -> [w1279] mode=indexing
                            tunnel: w1268 -> [w1280]
                            tunnel: [w1280] -> w1264
                            tunnel: [w1277] -> w1272 mode=indexing
                            n325 = Index Array(array=w1279, index=3) -> (element=w1277:string)
                          }
                          n326 = Unbundle By Name(w1264) -> ("status"=w1260:bool)
                        }
                      }
                      frame 1 {
                        n327 = for {
                          N: w1287 -> [_]
                          tunnel: w1285 -> [w1304]
                          tunnel: [w1300] -> w1281 mode=indexing
                          tunnel: w1286 -> [w1302]
                          tunnel: w1283 -> [w1290]
                          tunnel: [w1292] -> w1284
                          tunnel: w1282 -> [w1291]
                          i -> [w1299]
                          stop <- w1288 stop-if-true
                          n328 = Index Array(array=w1304, index=w1299) -> (element=w1303:string)
                          n329 = Index Array(array=w1302, index=w1299) -> (element=w1301:string)
                          n330 = call "WSVCAP SHL Host TL RFFE Write - Multiple DUTs - Common Data.vi"("Data Out"=w1303, "error in"=w1290, "Log (T)"=FALSE) -> ("error out"=w1294:errorcluster)  [unwired: 12 in]
                          n331 = local write "STATUS"(w1301) -> ()
                          n332 = call "Delay.vi"("milliseconds to wait"=u32 10, "error in (no error)"=w1294) -> ("error out"=w1298:errorcluster)  [unwired: 9 in]
                          n333 = call "WS1050 AD7747 READ 36 DUT.vi"("error in"=w1298, "Log (T)"=w1291, "DUT Mask Mode (All)"=WSVCAP_SHL_I2C_DUT_Mask_Mode_Enum."C1") -> ("error out"=w1296:errorcluster, "AD7747 Values"=w1297:string[][])  [unwired: 7 in]
                          n334 = for {
                            tunnel: w1297 -> [w1307] mode=indexing
                            tunnel: w1296 -> [w1308]
                            tunnel: [w1308] -> w1292
                            tunnel: [w1305] -> w1300 mode=indexing
                            n335 = Index Array(array=w1307, index=1) -> (element=w1305:string)
                          }
                          n336 = Unbundle By Name(w1292) -> ("status"=w1288:bool)
                        }
                      }
                    }
                  }
                  frame True {
                  }
                }
                n337 = Transpose 2D Array(2D array=w1222) -> (transposed array=w1231:string[][])
                "CAP_C2" <- w1231
              }
              frame #3 {
                n338 = Array Size(array=w1328) -> (size(s)=w1329:i32)
                n339 = case shown="True" w1311 {
                  tunnel: w1329 -> [w1346 _]
                  tunnel: w1328 -> [w1345 _]
                  tunnel: w1327 -> [w1344 _]
                  tunnel: w1322 -> [w1343 w1404]
                  tunnel: w1318 -> [w1342 _]
                  tunnel: [w1341 string[][] []] -> w1316
                  tunnel: w1315 -> [w1340 _]
                  tunnel: [w1339 w1404] -> w1314
                  frame False {
                    n340 = case shown="2" w1340 {
                      tunnel: w1346 -> [w1353 w1381]
                      tunnel: w1345 -> [w1352 w1380]
                      tunnel: w1344 -> [w1351 w1379]
                      tunnel: w1343 -> [w1350 w1378]
                      tunnel: [w1349 w1377] -> w1339
                      tunnel: w1342 -> [w1348 w1376]
                      tunnel: [w1347 w1375] -> w1341
                      frame 0, 1, Default {
                        n341 = for {
                          N: w1353 -> [_]
                          tunnel: w1351 -> [w1370]
                          tunnel: [w1366] -> w1347 mode=indexing
                          tunnel: w1352 -> [w1368]
                          tunnel: w1350 -> [w1356]
                          tunnel: [w1358] -> w1349
                          tunnel: w1348 -> [w1357]
                          i -> [w1365]
                          stop <- w1354 stop-if-true
                          n342 = Index Array(array=w1370, index=w1365) -> (element=w1369:string)
                          n343 = Index Array(array=w1368, index=w1365) -> (element=w1367:string)
                          n344 = local write "STATUS"(w1367) -> ()
                          n345 = call "WSVCAP SHL Host TL RFFE Write - Multiple DUTs - Common Data.vi"("Data Out"=w1369, "error in"=w1356, "Log (T)"=FALSE) -> ("error out"=w1360:errorcluster)  [unwired: 12 in]
                          n346 = call "Delay.vi"("milliseconds to wait"=u32 10, "error in (no error)"=w1360) -> ("error out"=w1364:errorcluster)  [unwired: 9 in]
                          n347 = call "WS1050 AD7747 READ 36 DUT.vi"("error in"=w1364, "Log (T)"=w1357, "DUT Mask Mode (All)"=WSVCAP_SHL_I2C_DUT_Mask_Mode_Enum."C3") -> ("error out"=w1362:errorcluster, "AD7747 Values"=w1363:string[][])  [unwired: 7 in]
                          n348 = for {
                            tunnel: w1363 -> [w1373] mode=indexing
                            tunnel: w1362 -> [w1374]
                            tunnel: [w1374] -> w1358
                            tunnel: [w1371] -> w1366 mode=indexing
                            n349 = Index Array(array=w1373, index=5) -> (element=w1371:string)
                          }
                          n350 = Unbundle By Name(w1358) -> ("status"=w1354:bool)
                        }
                      }
                      frame 2 {
                        n351 = for {
                          N: w1381 -> [_]
                          tunnel: w1379 -> [w1398]
                          tunnel: [w1394] -> w1375 mode=indexing
                          tunnel: w1380 -> [w1396]
                          tunnel: w1378 -> [w1384]
                          tunnel: [w1386] -> w1377
                          tunnel: w1376 -> [w1385]
                          i -> [w1393]
                          stop <- w1382 stop-if-true
                          n352 = Index Array(array=w1398, index=w1393) -> (element=w1397:string)
                          n353 = Index Array(array=w1396, index=w1393) -> (element=w1395:string)
                          n354 = local write "STATUS"(w1395) -> ()
                          n355 = call "WSVCAP SHL Host TL RFFE Write - Multiple DUTs - Common Data.vi"("Data Out"=w1397, "error in"=w1384, "Log (T)"=FALSE) -> ("error out"=w1388:errorcluster)  [unwired: 12 in]
                          n356 = call "Delay.vi"("milliseconds to wait"=u32 10, "error in (no error)"=w1388) -> ("error out"=w1392:errorcluster)  [unwired: 9 in]
                          n357 = call "WS1050 AD7747 READ 36 DUT.vi"("error in"=w1392, "Log (T)"=w1385, "DUT Mask Mode (All)"=WSVCAP_SHL_I2C_DUT_Mask_Mode_Enum."C1") -> ("error out"=w1390:errorcluster, "AD7747 Values"=w1391:string[][])  [unwired: 7 in]
                          n358 = for {
                            tunnel: w1391 -> [w1401] mode=indexing
                            tunnel: w1390 -> [w1402]
                            tunnel: [w1402] -> w1386
                            tunnel: [w1399] -> w1394 mode=indexing
                            n359 = Index Array(array=w1401, index=1) -> (element=w1399:string)
                          }
                          n360 = Unbundle By Name(w1386) -> ("status"=w1382:bool)
                        }
                      }
                    }
                  }
                  frame True {
                  }
                }
                n361 = Transpose 2D Array(2D array=w1316) -> (transposed array=w1323:string[][])
                "CAP_C3" <- w1323
              }
              frame #4 {
                # "VPI Testing @ 35V"
                n362 = call "WS1050 Delta C Calculation.vi"("error in (no error)"=w1446, "DCap Target(pF)"=w1445, "Input"=w1448) -> ("error out"=w1443:errorcluster, "Total Bank Delta C(pF)"=w1436:string[], "% Bank DeltaC"=w1440:string[])  [unwired: 3 in, 3 out]
                n363 = call "WS1050 Delta C Calculation.vi"("error in (no error)"=w1446, "DCap Target(pF)"=w1445, "Input"=w1447) -> ("error out"=w1444:errorcluster, "Total Bank Delta C(pF)"=w1435:string[], "% Bank DeltaC"=w1438:string[])  [unwired: 3 in, 3 out]
                n364 = call "WS1050 Delta C Calculation.vi"("error in (no error)"=w1446, "DCap Target(pF)"=w1445, "Input"=w1439) -> ("error out"=w1442:errorcluster, "Total Bank Delta C(pF)"=w1434:string[], "% Bank DeltaC"=w1437:string[])  [unwired: 3 in, 3 out]
                n365 = Merge Errors(w1443, w1444, w1442) -> (w1441:errorcluster)
                n366 = case shown="1, Default" w1449 {
                  tunnel: w1441 -> [w1647 w1655]
                  tunnel: [w1647 w1655] -> w1408
                  tunnel: w1440 -> [w1643 w1651]
                  tunnel: w1438 -> [w1642 w1650]
                  tunnel: w1437 -> [w1641 w1649]
                  tunnel: w1436 -> [w1646 w1654]
                  tunnel: [w1646 w1654] -> w1433
                  tunnel: w1435 -> [w1645 w1653]
                  tunnel: [w1645 w1653] -> w1432
                  tunnel: w1434 -> [w1644 w1652]
                  tunnel: [w1644 w1652] -> w1431
                  frame 0 {
                    n367 = Build Array(w1643, w1642, w1641) -> (→"% Delta C_T0":string[][])
                  }
                  frame 1, Default {
                    n368 = Build Array(w1651, w1650, w1649) -> (→"% Delta C":string[][])
                  }
                }
                "Total Delta C1(pF)" <- w1433
                "Total Delta C2(pF)" <- w1432
                "Total Delta C3(pF)" <- w1431
                n369 = call "WS1050_51 VPI Header.vi"("VPI Name"="VPI Name", "VPI_Cmd"="VPI_Cmd", "Cmin/Act"=w1406, "WS1050/51"=w1417, "error in (no error)"=w1418) -> ("VPI_1"=w1416:string[], "VPI_2"=w1414:string[], "VPI Header"=w1415:string[], "VPI_3"=w1413:string[], "Cmd_3"=w1410:string[], "Cmd_1"=w1412:string[], "Cmd_2"=w1411:string[], "error out"=w1409:errorcluster)  [unwired: 3 in]
                n370 = Merge Errors(w1409, w1408) -> (w1407:errorcluster)
                n371 = case shown="False" w1405 {
                  tunnel: [w1476 w1631] -> w1461
                  tunnel: [w1475 w1631] -> w1460
                  tunnel: w1456 -> [w1474 w1629]
                  tunnel: [w1473 w1629] -> w1455
                  tunnel: [w1472 w1631] -> w1452
                  tunnel: [w1471 "" ("Data Out")] -> w1429
                  tunnel: [w1470 w1630] -> w1427
                  tunnel: w1423 -> [w1469 _]
                  tunnel: w1416 -> [w1468 _]
                  tunnel: w1414 -> [w1467 _]
                  tunnel: w1413 -> [w1466 _]
                  tunnel: w1412 -> [w1465 _]
                  tunnel: w1411 -> [w1464 _]
                  tunnel: w1410 -> [w1463 _]
                  tunnel: w1407 -> [w1462 w1630]
                  frame False {
                    n372 = case shown="False" w1469 {
                      tunnel: [w1479 w1500] -> w1470
                      tunnel: [w1477 w1518] -> w1476
                      tunnel: [w1477 w1504] -> w1475
                      tunnel: w1474 -> [w1484 w1517]
                      tunnel: [w1484 w1517] -> w1473
                      tunnel: w1465 -> [_ w1516]
                      tunnel: w1464 -> [_ w1510]
                      tunnel: w1463 -> [_ w1506]
                      tunnel: [w1477 w1515] -> w1472
                      tunnel: w1468 -> [w1482 w1513]
                      tunnel: w1467 -> [_ w1511]
                      tunnel: w1466 -> [_ w1507]
                      tunnel: ["NA" ("string") w1494] -> w1471
                      tunnel: w1462 -> [w1480 w1498]
                      frame False {
                        n373 = Array Size(array=w1482) -> (size(s)=w1481:i32)
                        n374 = for {
                          N: w1481 -> [_]
                          tunnel: [w1486] -> w1478 mode=indexing
                          tunnel: w1480 -> [w1485]
                          tunnel: [w1485] -> w1479
                          n375 = for {
                            N: 36 -> [_]
                            tunnel: [""] -> w1486 mode=indexing
                          }
                        }
                        n376 = Transpose 2D Array(2D array=w1478) -> (transposed array=w1477:string[][])
                        n377 = local write "VPI C1"(w1477) -> ()
                        n378 = local write "VPI C2"(w1477) -> ()
                        n379 = local write "VPI C3"(w1477) -> ()
                      }
                      frame True {
                        w1499 = FALSE ("Log (T)")
                        # "Set CP VPI"
                        n380 = call "WSVCAP SHL Host TL RFFE Write - Multiple DUTs - Common Data.vi"("Data Out"="074820", "error in"=w1498, "Log (T)"=w1499) -> ("error out"=w1496:errorcluster)  [unwired: 12 in]
                        n381 = call "Delay.vi"("milliseconds to wait"=u32 10, "error in (no error)"=w1496) -> ("error out"=w1492:errorcluster)  [unwired: 9 in]
                        n382 = case shown="0, Default" "CP VPI" {
                          selector: "CP VPI" -> [w1523 w1528 w1533 w1538 w1543 w1548 w1553 w1558 w1562]
                          tunnel: string[] ["07476F", "074776", "074765", "074769", "07477B", "07477C", "07477D", "074779", "07476B"] -> [w1524 w1529 w1534 w1539 w1544 w1549 w1554 w1559 w1564]
                          tunnel: [w1522 w1527 w1532 w1537 w1542 w1547 w1552 w1557 w1563] -> w1491
                          tunnel: ["35.0" ("Data Out") "27.5" ("Data Out") "30.5" ("Data Out") "44.0" ("Data Out") "50.0" ("Data Out") "55.0" ("Data Out") "42.5" ("Data Out") "32.0" ("Data Out") "40.25" ("Data Out")] -> w1494
                          tunnel: [w1520 w1525 w1530 w1535 w1540 w1545 w1550 w1555 w1560] -> w1493
                          tunnel: w1492 -> [w1520 w1525 w1530 w1535 w1540 w1545 w1550 w1555 w1560]
                          frame 0, Default {
                            n383 = Index Array(array=w1524, index=w1523) -> (element=w1522:string)
                          }
                          frame 2 {
                            n384 = Index Array(array=w1529, index=w1528) -> (element=w1527:string)
                          }
                          frame 3 {
                            n385 = Index Array(array=w1534, index=w1533) -> (element=w1532:string)
                          }
                          frame 4 {
                            n386 = Index Array(array=w1539, index=w1538) -> (element=w1537:string)
                          }
                          frame 5 {
                            n387 = Index Array(array=w1544, index=w1543) -> (element=w1542:string)
                          }
                          frame 6 {
                            n388 = Index Array(array=w1549, index=w1548) -> (element=w1547:string)
                          }
                          frame 7 {
                            n389 = Index Array(array=w1554, index=w1553) -> (element=w1552:string)
                          }
                          frame 8 {
                            n390 = Index Array(array=w1559, index=w1558) -> (element=w1557:string)
                          }
                          frame 1 {
                            n391 = Index Array(array=w1564, index=w1562) -> (element=w1563:string)
                          }
                        }
                        n392 = Array Size(array=w1513) -> (size(s)=w1519:i32)
                        n393 = call "WSVCAP SHL Host TL RFFE Write - Multiple DUTs - Common Data.vi"("Data Out"=w1491, "error in"=w1493, "Log (T)"=w1499) -> ("error out"=w1503:errorcluster)  [unwired: 12 in]
                        n394 = for {
                          N: w1519 -> [_]
                          tunnel: w1516 -> [w1623]
                          tunnel: [w1621] -> w1514 mode=indexing
                          tunnel: w1513 -> [w1620]
                          tunnel: w1503 -> [w1609]
                          tunnel: [w1611] -> w1502
                          i -> [w1619]
                          stop <- w1607 stop-if-true
                          n395 = Index Array(array=w1623, index=w1619) -> (element=w1622:string)
                          n396 = Index Array(array=w1620, index=w1619) -> (element=w1618:string)
                          n397 = local write "STATUS"(w1618) -> ()
                          n398 = call "WSVCAP SHL Host TL RFFE Write - Multiple DUTs - Common Data.vi"("Data Out"=w1622, "error in"=w1609, "Log (T)"=FALSE) -> ("error out"=w1617:errorcluster)  [unwired: 12 in]
                          n399 = call "Delay.vi"("milliseconds to wait"=u32 10, "error in (no error)"=w1617) -> ("error out"=w1613:errorcluster)  [unwired: 9 in]
                          n400 = call "WS1050 AD7747 READ 36 DUT.vi"("error in"=w1613, "Log (T)"=FALSE, "DUT Mask Mode (All)"=WSVCAP_SHL_I2C_DUT_Mask_Mode_Enum."C1") -> ("error out"=w1615:errorcluster, "AD7747 Values"=w1614:string[][])  [unwired: 7 in]
                          n401 = for {
                            tunnel: [w1626] -> w1621 mode=indexing
                            tunnel: w1615 -> [w1625]
                            tunnel: [w1625] -> w1611
                            tunnel: w1614 -> [w1624] mode=indexing
                            n402 = Index Array(array=w1624, index=1) -> (element=w1626:string)
                          }
                          n403 = Unbundle By Name(w1611) -> ("status"=w1607:bool)
                        }
                        n404 = Transpose 2D Array(2D array=w1514) -> (transposed array=w1518:string[][])
                        "VPI C1" <- w1518
                        n405 = Array Size(array=w1511) -> (size(s)=w1512:i32)
                        n406 = for {
                          N: w1512 -> [_]
                          tunnel: w1510 -> [w1602]
                          tunnel: [w1600] -> w1509 mode=indexing
                          tunnel: w1511 -> [w1599]
                          tunnel: w1502 -> [w1588]
                          tunnel: [w1590] -> w1501
                          i -> [w1598]
                          stop <- w1586 stop-if-true
                          n407 = Index Array(array=w1602, index=w1598) -> (element=w1601:string)
                          n408 = Index Array(array=w1599, index=w1598) -> (element=w1597:string)
                          n409 = call "WSVCAP SHL Host TL RFFE Write - Multiple DUTs - Common Data.vi"("Data Out"=w1601, "error in"=w1588, "Log (T)"=FALSE) -> ("error out"=w1596:errorcluster)  [unwired: 12 in]
                          n410 = local write "STATUS"(w1597) -> ()
                          n411 = call "Delay.vi"("milliseconds to wait"=u32 10, "error in (no error)"=w1596) -> ("error out"=w1592:errorcluster)  [unwired: 9 in]
                          n412 = call "WS1050 AD7747 READ 36 DUT.vi"("error in"=w1592, "Log (T)"=FALSE, "DUT Mask Mode (All)"=WSVCAP_SHL_I2C_DUT_Mask_Mode_Enum."C2") -> ("error out"=w1594:errorcluster, "AD7747 Values"=w1593:string[][])  [unwired: 7 in]
                          n413 = for {
                            tunnel: [w1605] -> w1600 mode=indexing
                            tunnel: w1594 -> [w1604]
                            tunnel: [w1604] -> w1590
                            tunnel: w1593 -> [w1603] mode=indexing
                            n414 = Index Array(array=w1603, index=3) -> (element=w1605:string)
                          }
                          n415 = Unbundle By Name(w1590) -> ("status"=w1586:bool)
                        }
                        n416 = Transpose 2D Array(2D array=w1509) -> (transposed array=w1515:string[][])
                        "VPI C2" <- w1515
                        n417 = Array Size(array=w1507) -> (size(s)=w1508:i32)
                        n418 = for {
                          N: w1508 -> [_]
                          tunnel: w1506 -> [w1581]
                          tunnel: [w1579] -> w1505 mode=indexing
                          tunnel: w1507 -> [w1578]
                          tunnel: w1501 -> [w1567]
                          tunnel: [w1569] -> w1500
                          i -> [w1577]
                          stop <- w1565 stop-if-true
                          n419 = Index Array(array=w1581, index=w1577) -> (element=w1580:string)
                          n420 = Index Array(array=w1578, index=w1577) -> (element=w1576:string)
                          n421 = call "WSVCAP SHL Host TL RFFE Write - Multiple DUTs - Common Data.vi"("Data Out"=w1580, "error in"=w1567, "Log (T)"=FALSE) -> ("error out"=w1575:errorcluster)  [unwired: 12 in]
                          n422 = local write "STATUS"(w1576) -> ()
                          n423 = call "Delay.vi"("milliseconds to wait"=u32 10, "error in (no error)"=w1575) -> ("error out"=w1571:errorcluster)  [unwired: 9 in]
                          n424 = call "WS1050 AD7747 READ 36 DUT.vi"("error in"=w1571, "Log (T)"=FALSE, "DUT Mask Mode (All)"=WSVCAP_SHL_I2C_DUT_Mask_Mode_Enum."C3") -> ("error out"=w1573:errorcluster, "AD7747 Values"=w1572:string[][])  [unwired: 7 in]
                          n425 = for {
                            tunnel: [w1584] -> w1579 mode=indexing
                            tunnel: w1573 -> [w1583]
                            tunnel: [w1583] -> w1569
                            tunnel: w1572 -> [w1582] mode=indexing
                            n426 = Index Array(array=w1582, index=5) -> (element=w1584:string)
                          }
                          n427 = Unbundle By Name(w1569) -> ("status"=w1565:bool)
                        }
                        n428 = Transpose 2D Array(2D array=w1505) -> (transposed array=w1504:string[][])
                        "VPI C3" <- w1504
                      }
                    }
                  }
                  frame True {
                    w1631 = string[][] []
                  }
                }
                n429 = Insert Into Array(array=w1451, new element=w1415) -> (w1450:string[])  [unwired: 1 in]
                n430 = case shown="True" w1428 {
                  tunnel: w1427 -> [w1633 w1638]
                  tunnel: [w1634 w1637] -> w1426
                  frame False {
                    n431 = call "WSVCAP SHL Host TL RFFE Write - Multiple DUTs - Common Data.vi"("Data Out"="074820", "error in"=w1633, "Log (T)"=FALSE) -> ("error out"=w1634:errorcluster)  [unwired: 12 in]
                  }
                  frame True {
                    n432 = call "WSVCAP SHL Host TL RFFE Write - Multiple DUTs - Common Data.vi"("Data Out"="074800", "error in"=w1638, "Log (T)"=FALSE) -> ("error out"=w1637:errorcluster)  [unwired: 12 in]
                  }
                }
                n433 = call "Delay.vi"("milliseconds to wait"=u32 10, "error in (no error)"=w1426) -> ("error out"=w1425:errorcluster)  [unwired: 9 in]
              }
              frame #5 {
                # "VSA Testing"
                n434 = case shown="True" w1656 {
                  tunnel: w1696 -> [w1706 w1776]
                  tunnel: w1687 -> [w1705 w1775]
                  tunnel: [w1704 w1775] -> w1686
                  tunnel: [w1703 string[][] []] -> w1676
                  tunnel: [w1702 w1777] -> w1675
                  tunnel: [w1701 w1777] -> w1672
                  tunnel: [w1700 w1776] -> w1670
                  tunnel: [w1699 w1777] -> w1669
                  tunnel: w1657 -> [w1698 _]
                  frame False {
                    n435 = case shown="True" w1698 {
                      tunnel: w1706 -> [w1708 w1722]
                      tunnel: [w1707 w1721] -> w1700
                      tunnel: [w1712 w1728] -> w1704
                      tunnel: w1705 -> [w1712 w1727]
                      tunnel: [w1709 w1725] -> w1702
                      tunnel: [w1709 w1724] -> w1701
                      tunnel: [w1709 w1723] -> w1699
                      tunnel: [w1710 w1726] -> w1703
                      frame False {
                        n436 = for {
                          tunnel: dbl[] [0.0, 0.0, 0.0] -> [w1717] mode=indexing
                          tunnel: [w1716] -> w1710 mode=indexing
                          tunnel: [w1713] -> w1709 mode=indexing
                          tunnel: w1708 -> [w1714]
                          tunnel: [w1714] -> w1707
                          n437 = Number To Fractional String(number=w1717) -> (F-format string=w1718:string)  [unwired: 3 in]
                          n438 = for {
                            N: 36 -> [_]
                            tunnel: w1718 -> [w1720]
                            tunnel: [w1720] -> w1716 mode=indexing
                            tunnel: [""] -> w1713 mode=indexing
                          }
                        }
                      }
                      frame True {
                        n439 = for {
                          tunnel: "VSA Voltage(V)" -> [w1752] mode=indexing
                          tunnel: [w1756] -> w1728
                          tunnel: w1727 -> [w1754]
                          tunnel: [w1753] -> w1725 mode=indexing
                          tunnel: [w1740] -> w1724 mode=indexing
                          tunnel: [w1749] -> w1726 mode=indexing
                          tunnel: [w1734] -> w1723 mode=indexing
                          tunnel: w1722 -> [w1733]
                          tunnel: [w1732] -> w1721
                          w1731 = FALSE ("Log (T)")
                          w1748 = u16 0 items=["Voltage", "Current"] ("Source Mode  (0: Voltage)")
                          n440 = call "Ke2400 Configure Output.vi"("Source Mode  (0: Voltage)"=w1748, "error in (no error)"=w1733, "Compliance  Level (0.1)"=0.1, "Output Level (0)"=w1752, "VISA resource name"=w1754) -> ("error out"=w1760:errorcluster, "VISA resource name out"=w1758:refnum<visa-resource-name>)  [unwired: 5 in]
                          n441 = Number To Fractional String(number=w1752) -> (F-format string=w1751:string)  [unwired: 3 in]
                          n442 = call "Ke2400 Enable.vi"("error in (no error)"=w1760, "ON/OFF"=TRUE ("Enable Output (T: Enable)"), "VISA resource name"=w1758) -> ("error out"=w1761:errorcluster, "VISA resource name out"=w1756:refnum<visa-resource-name>)  [unwired: 7 in]
                          n443 = call "Delay.vi"("milliseconds to wait"=u32 10, "error in (no error)"=w1761) -> ("error out"=w1747:errorcluster)  [unwired: 9 in]
                          n444 = call "WS1050 AD7747 READ 36 DUT.vi"("error in"=w1747, "Log (T)"=w1731, "DUT Mask Mode (All)"=WSVCAP_SHL_I2C_DUT_Mask_Mode_Enum."C1") -> ("error out"=w1744:errorcluster, "AD7747 Values"=w1746:string[][])  [unwired: 7 in]
                          n445 = for {
                            tunnel: w1746 -> [w1772] mode=indexing
                            tunnel: [w1773] -> w1753 mode=indexing
                            tunnel: w1744 -> [w1771]
                            tunnel: [w1771] -> w1743
                            n446 = Index Array(array=w1772, index=1) -> (element=w1773:string)
                          }
                          n447 = for {
                            N: 36 -> [_]
                            tunnel: w1751 -> [w1770]
                            tunnel: [w1770] -> w1749 mode=indexing
                          }
                          n448 = call "WS1050 AD7747 READ 36 DUT.vi"("error in"=w1743, "Log (T)"=w1731, "DUT Mask Mode (All)"=WSVCAP_SHL_I2C_DUT_Mask_Mode_Enum."C2") -> ("error out"=w1741:errorcluster, "AD7747 Values"=w1739:string[][])  [unwired: 7 in]
                          n449 = for {
                            tunnel: w1739 -> [w1767] mode=indexing
                            tunnel: [w1768] -> w1740 mode=indexing
                            tunnel: w1741 -> [w1766]
                            tunnel: [w1766] -> w1738
                            n450 = Index Array(array=w1767, index=3) -> (element=w1768:string)
                          }
                          n451 = call "WS1050 AD7747 READ 36 DUT.vi"("error in"=w1738, "Log (T)"=w1731, "DUT Mask Mode (All)"=WSVCAP_SHL_I2C_DUT_Mask_Mode_Enum."C3") -> ("error out"=w1736:errorcluster, "AD7747 Values"=w1735:string[][])  [unwired: 7 in]
                          n452 = local write "STATUS"("VSA Testing...." ("STATUS")) -> ()
                          n453 = for {
                            tunnel: w1735 -> [w1763] mode=indexing
                            tunnel: [w1764] -> w1734 mode=indexing
                            tunnel: w1736 -> [w1762]
                            tunnel: [w1762] -> w1732
                            n454 = Index Array(array=w1763, index=5) -> (element=w1764:string)
                          }
                        }
                      }
                    }
                  }
                  frame True {
                    w1777 = string[][] []
                  }
                }
                n455 = Transpose 2D Array(2D array=w1676) -> (transposed array=w1674:string[][])
                n456 = Transpose 2D Array(2D array=w1675) -> (transposed array=w1673:string[][])
                n457 = Transpose 2D Array(2D array=w1672) -> (transposed array=w1671:string[][])
                n458 = Transpose 2D Array(2D array=w1669) -> (transposed array=w1668:string[][])
                n459 = call "WS1050_VSA_Convert_Data.vi"("VSA_C3"=w1668, "error in (no error)"=w1670, "VSA_C2"=w1671, "VSA_C1"=w1673, "Voltage"=w1674) -> ("error out"=w1667:errorcluster, "VSA_V3"=w1664:string[][], "VSA_V2"=w1665:string[][], "VSA_V1"=w1666:string[][])  [unwired: 3 in]
                "VSA_V1" <- w1666
                "VSA_V2" <- w1665
                "VSA_V3" <- w1664
                n460 = case shown="True" w1657 {
                  tunnel: w1686 -> [w1780 w1786]
                  tunnel: [w1780 w1785] -> w1685
                  tunnel: w1667 -> [w1779 w1784]
                  tunnel: [w1779 w1781] -> w1684
                  frame False {
                  }
                  frame True {
                    w1782 = u16 0 items=["Voltage", "Current"] ("Source Mode  (0: Voltage)")
                    n461 = call "Ke2400 Configure Output.vi"("Source Mode  (0: Voltage)"=w1782, "error in (no error)"=w1784, "Output Level (0)"=0.0, "VISA resource name"=w1786) -> ("error out"=w1781:errorcluster, "VISA resource name out"=w1785:refnum<visa-resource-name>)  [unwired: 6 in]
                  }
                }
                n462 = call "Delay.vi"("milliseconds to wait"=u32 50, "error in (no error)"=w1684) -> ("error out"=w1683:errorcluster)  [unwired: 9 in]
              }
              frame #6 {
                # "Handshake Check and EFuse Readback"
                n463 = Or(x=w1795, y=w1805) -> (x .or. y?=w1804:bool)
                n464 = Add(x=w1817, y=w1816) -> (x+y=w1803:u64)
                n465 = case shown="False" w1804 {
                  tunnel: w1830 -> [w1843 _]
                  tunnel: w1829 -> [w1842 w1848]
                  tunnel: [w1841 w1848] -> w1828
                  tunnel: w1827 -> [w1840 _]
                  tunnel: w1826 -> [w1839 _]
                  tunnel: w1825 -> [w1838 _]
                  tunnel: [w1834 w1847] -> w1824
                  tunnel: [w1833 w1847] -> w1819
                  tunnel: w1803 -> [w1832 _]
                  tunnel: w1810 -> [w1831 _]
                  frame False {
                    n466 = call "WS1050_36DUT_Handshake Check R1_Record All Regs Ver1.0.vi"("file path (use dialog)"=w1843, "Reg1_Bit Cntrl"="Reg1_Bit Cntrl", "File Name"=w1831, "SN"=w1838, "Loop"=w1832, "error"=w1842, "Lot #"=w1840, "Wafer #"=w1839) -> ("Pass/Fail"=→"EFuse Readback Status":bool[], "EFuse Read back"=w1833:string[], "Status"=w1834:string[], "error out"=w1841:errorcluster)  [unwired: 6 in, 2 out]
                    n467 = case shown="1, Default" w1832 {
                      tunnel: w1833 -> [w1844 w1845]
                      frame 0 {
                        "EFuse RB T0" <- w1844
                      }
                      frame 1, Default {
                        "Current EFuse Read back" <- w1845
                      }
                    }
                    n468 = local write "STATUS"("Hand Shake & EFuse Readback...." ("STATUS")) -> ()
                  }
                  frame True {
                    n469 = for {
                      N: 36 -> [_]
                      tunnel: [""] -> w1847 mode=indexing
                    }
                  }
                }
                n470 = Add(x=w1803, y=w1800) -> (x+y=w1801:u64)
                "TTCompleted" <- w1801
                n471 = Number To Engineering String(4:w1801) -> (0:w1815:string)  [unwired: 3 in]
                n472 = Build Array(w1814, w1812, w1811) -> (w1813:string[])
              }
              frame #7 {
                # "Save Data"
                n473 = Increment(x=w1862) -> (x+1=w1861:i32)
                n474 = Multiply(x=w1861, y=36) -> (x*y=w1856:i32)
                n475 = Path To String(path=w1866) -> (string=w1865:string)
                n476 = Bundle("Test Program"=w1897, "Comment"=w1896, "Data Out"=w1873, "Data Out"=w1872, "Data Out"=w1871, w1870, "Data Out"=w1869, "Data Out"=w1868, "Data Out"=w1867, "Freq(Hz)"=w1854, "Board#"=w1852) -> (w1853:T8)  [unwired: 1 in]
                n477 = case shown="False" w1851 {
                  tunnel: w1902 -> [w1929 w1931]
                  tunnel: [w1928 w1931] -> w1901
                  tunnel: w1900 -> [w1927 _]
                  tunnel: w1899 -> [w1926 _]
                  tunnel: w1898 -> [w1925 _]
                  tunnel: w1895 -> [w1924 _]
                  tunnel: w1893 -> [w1923 _]
                  tunnel: w1892 -> [w1922 _]
                  tunnel: w1891 -> [w1921 _]
                  tunnel: w1890 -> [w1920 _]
                  tunnel: w1889 -> [w1919 _]
                  tunnel: w1886 -> [w1918 _]
                  tunnel: w1885 -> [w1917 _]
                  tunnel: w1884 -> [w1916 _]
                  tunnel: w1882 -> [w1915 _]
                  tunnel: w1881 -> [w1914 _]
                  tunnel: w1880 -> [w1913 _]
                  tunnel: w1879 -> [w1912 _]
                  tunnel: w1878 -> [w1911 _]
                  tunnel: w1877 -> [w1910 _]
                  tunnel: w1876 -> [w1909 _]
                  tunnel: w1875 -> [w1908 _]
                  tunnel: w1874 -> [w1907 _]
                  tunnel: w1866 -> [w1906 _]
                  tunnel: w1859 -> [w1905 _]
                  tunnel: w1853 -> [w1904 _]
                  tunnel: ["Save Data...." ("STATUS") "Stop test..." ("STATUS")] -> w1850
                  frame False {
                    n478 = call "WS1050_36 DUT SData Ver1.0.vi"("TMN DC\\CAP Data Log File Path"=w1906, "Lot#"=w1926, "Total Delta C1(pF)"=w1909, "VSA_V1"=w1917, "Wafer#"=w1924, "File Name"=w1905, "Total Delta C2(pF)"=w1908, "error in"=w1929, "TP/Comment"=w1904, "EFuse"=w1920, "Data Output C3"=w1911, "Temperature"=w1915, "VSA_V2"=w1918, "VPI C3"=w1913, "Data Output C1"=w1923, "VPI C2"=w1912, "SN"=w1927, "R/W Status"=w1925, "Cap Header"=w1914, "HD/Cycles Completed"=w1919, "Data Output C2"=w1910, "VSA_V3"=w1916, "Current"=w1922, "VPI C1"=w1921, "Total Delta C3(pF)"=w1907) -> ("error out"=w1928:errorcluster)  [unwired: 2 in]
                  }
                  frame True {
                  }
                }
                n479 = case shown="True" "Debug" {
                  tunnel: w1856 -> [w1932 w1935]
                  tunnel: [w1932 w1933] -> w1855
                  frame False {
                  }
                  frame True {
                    n480 = Multiply(x=w1935, y="No of Rows\nFrom Spread Sheet") -> (x*y=w1933:i32)
                  }
                }
                n481 = Concatenate Strings(w1865, "\\" ("string"), w1859, "_Multi Socket Data.csv" ("string")) -> (w1864:string)
                n482 = local write "STATUS"(w1850) -> ()
              }
              frame #8 {
                n483 = case shown="True" "Plot Delta Cmin" {
                  tunnel: w1941 -> [w1955 w1970]
                  tunnel: [w1955 w1966] -> w1940
                  tunnel: w1939 -> [_ w1962]
                  tunnel: w1937 -> [_ w1960]
                  frame False {
                  }
                  frame True {
                    n484 = String To Path(string=w1962) -> (path=w1961:path)
                    n485 = call "Delay.vi"("milliseconds to wait"=u32 50, "error in (no error)"=w1970) -> ("error out"=w1969:errorcluster)  [unwired: 9 in]
                    n486 = call "36DUT Plot From Spread Sheet.vi"("Plot"="Plot", "No of Rows"=w1960, "error in (no error)"=w1969, "Bank"="Bank C1", "file path (dialog if empty)"=w1961) -> ("error out"=w1964:errorcluster, "Delta C_Min Plot"=→"Min Plot_1":dbl[][])  [unwired: 5 in]
                    n487 = call "36DUT Plot From Spread Sheet.vi"("Plot"="Plot", "No of Rows"=w1960, "error in (no error)"=w1964, "Bank"="Bank C2", "file path (dialog if empty)"=w1961) -> ("error out"=w1965:errorcluster, "Delta C_Min Plot"=→"Min Plot_2":dbl[][])  [unwired: 5 in]
                    n488 = call "36DUT Plot From Spread Sheet.vi"("Plot"="Plot", "No of Rows"=w1960, "error in (no error)"=w1965, "Bank"="Bank C3", "file path (dialog if empty)"=w1961) -> ("error out"=w1966:errorcluster, "Delta C_Min Plot"=→"Min Plot_3":dbl[][])  [unwired: 5 in]
                  }
                }
                n489 = Get Date/Time In Seconds() -> (seconds since 1Jan1904=w1948:timestamp)
                n490 = Get Date/Time String(seconds (now)=w1948, want seconds? (F)=TRUE) -> (date string=→"date string":string, time string=→"Previous Time":string)  [unwired: 1 in]
                n491 = Greater Or Equal?(x=w1945, y="Set HD/Cycle \nto Complete") -> (x >= y?=w1952:bool)
                n492 = Greater Or Equal?(x=w1944, y="TTF Completed") -> (x >= y?=w1943:bool)
                "No of HD/Cycle\nCompleted" <- w1945
              }
            }
            n493 = Increment(x=w591) -> (x+1=→"Loop \ncompleted":i32)
            n494 = call "Delay.vi"("milliseconds to wait"=u32 10, "error in (no error)"=w483) -> ("error out"=w484:errorcluster)  [unwired: 9 in]
            n495 = Compound Arithmetic op=OR(w660, w561, w587) -> (w600:bool)
          }
          "Total Time" <- w421
          n496 = Increment(x=w419) -> (x+1=→"Run Loops":i32)
          n497 = local write "No of HD/Cycle\nCompleted"(u64 0 ("No of HD/Cycle\nCompleted")) -> ()
          n498 = Unbundle By Name(w411) -> ("status"=w425:bool)
          n499 = Compound Arithmetic op=OR(w425, w417, w416) -> (w400:bool)
        }
        n500 = flat-sequence {
          tunnel: w280 -> [w339]
          tunnel: [w339] -> w279
          tunnel: [w338] -> w278
          tunnel: w277 -> [w338]
          frame #0 {
            n501 = One Button Dialog(message="Done!") -> ()  [unwired: 1 in, 1 out]
            n502 = local write "STATUS"("Completed!" ("STATUS")) -> ()
          }
        }
        n503 = for {
          tunnel: w302 -> [w1982]
          tunnel: w286 -> [w1981]
          tunnel: w331 -> [w1979] mode=indexing
          tunnel: [w1974] -> w301
          tunnel: [w1978] -> w330
          n504 = call "E3631A_Voltage Controller updated.vi"("VISA resource name"=w1981, "I_VDD(A)"=0.5, "Channel Controller"=w1979, "Voltage 1"=0.0, "Voltage 2"=3.3, "error in (no error)"=w1982, "I_3.3V (A)"=0.5) -> ("VISA resource name out"=w1978:refnum<visa-resource-name>, "error out"=w1975:errorcluster)  [unwired: 7 in]
          n505 = call "Delay.vi"("milliseconds to wait"=u32 100, "error in (no error)"=w1975) -> ("error out"=w1974:errorcluster)  [unwired: 9 in]
        }
        n506 = VISA Write(VISA resource name=w321, write buffer="SOUR:FUNC VOLT;VOLT:MODE FIX;RANG 100;LEV 0.0;:SENS:FUNC \"CURR\";CURR:PROT 60E-3;RANG 100E-3;:OUTP ON", error in (no error)=w302) -> (VISA resource name out=w319:refnum<visa-resource-name>, error out=w280:errorcluster)  [unwired: 1 out]
        n507 = Merge Errors(w301, w279) -> (w320:errorcluster)
      }
      frame True {
      }
    }
    n508 = Wait Until Next ms Multiple(millisecond multiple=u32 100) -> ()  [unwired: 1 out]
    n509 = Unbundle By Name(w66) -> ("status"=w65:bool)
    n510 = Compound Arithmetic op=OR(w64, w65, w86) -> (w94:bool)
    "STATUS" <- "Idle...." ("STATUS")
  }
  "Ke2000 Out" <- w10
  n511 = local write "stop During HD/Cycles"(w16) -> ()
  n512 = local write "stop"(w16) -> ()
  n513 = case shown="True" w25 {
    tunnel: [w2000 w2003] -> w8
    tunnel: w4 -> [w2000 w2002]
    frame False {
    }
    frame True {
      n514 = local write "Online"(FALSE ("Online")) -> ()
      n515 = call "WSVCAP SHL Host TL Close.vi"("error in"=w2002) -> ("error out"=w2003:errorcluster)  [unwired: 14 in]
    }
  }
  "error out" <- w8
  n516 = VISA Write(VISA resource name=w20, write buffer="SOUR:FUNC VOLT;VOLT:MODE FIX;RANG 100;LEV 0.0;:SENS:FUNC \"CURR\";CURR:PROT 60E-3;RANG 100E-3;:OUTP OFF", error in (no error)=w4) -> (VISA resource name out=→"VISA resource name out":refnum<visa-resource-name>, error out=w7:errorcluster)  [unwired: 1 out]
  n517 = VISA Write(VISA resource name=w5, write buffer=":INST:NSEL 1; :VOLT 0.000000;:OUTP 1;", error in (no error)=w4) -> (VISA resource name out=→"PS1 Out":refnum<visa-resource-name>, error out=w3:errorcluster)  [unwired: 1 out]
  n518 = Merge Errors(w3, w8, w7) -> (→"error out 2":errorcluster)
